vi "main 1.0.vi"() -> ()   [LabVIEW 2020]
uses:
  subvi/Newport ESP301/Newport ESP301.lvlib
  subvi/sp_manip.llb/sp_manip_lib.lvlib
  subvi/sp_manip.llb/tcp_gateway.lvlib
  subvi/PHOIBOS/DEFINITIONS/DEF_dev_type.ctl
  subvi/PHOIBOS/DEFINITIONS/DEF_dev_state.ctl
  <vilib>/Utility/file.llb/Write Delimited Spreadsheet (DBL).vi
  <vilib>/Analysis/NI_AALBase.lvlib
  <vilib>/Analysis/1siggen.llb/Ramp Pattern by Samples.vi
  <vilib>/Analysis/NI_AALPro.lvlib
  <vilib>/Analysis/_algsub.llb/Real Vector Norm.vi
  subvi/ZaberTSeries/ZaberTSeries.lvlib
  <vilib>/DAQmx/create/channels.llb/DAQmx Create Channel (DI-Digital Input).vi
  <vilib>/Utility/file.llb/Read Delimited Spreadsheet (string).vi
  <vilib>/Utility/file.llb/Write Delimited Spreadsheet (string).vi
panel:
  out "Pics L":i32=100
  out "Waveform Chart":dbl(graph)
  out "G2 X":cluster{dbl[], "Ramp Pattern":dbl[]}(graph)
  in  "reset every n pics":bool
  in  "pics2avg":i32=50
  in  "abort acq.":bool
  out "G2 Y":cluster{dbl[], "Ramp Pattern":dbl[]}(graph)={[0.0, 0.0, 0.0, 0.0, 0.0, 0.0, 0.0, 0.0, 0.0, 0.0, 0.0, 0.0, 0.0, 0.0, 0.0, 0.0, 0.0, 0.0, 0.0, 0.0, 0.0, 0.0, 0.0, 0.0, 0.0, 0.0, 0.0, 0.0, 0.0, 0.0, 0.0, 0.0, 0.0, 0.0, 0.0, 0.0, 0.0, 0.0, 0.0, 0.0, 0.0, 0.0, 0.0, 0.0, 0.0, 0.0, 0.0, 0.0, 0.0, 0.0, 0.0, 0.0, 0.0, 0.0, 0.0, 0.0, 0.0, 0.0, 0.0, 0.0, 0.0, 0.0, 0.0, 0.0, 0.0, 0.0, 0.0, 0.0, 0.0, 0.0, 0.0, 0.0, 0.0, 0.0, 0.0, 0.0, 0.0, 0.0, 0.0, 0.0, 0.0, 0.0, 0.0, 0.0, 0.0, 0.0, 0.0, 0.0, 0.0, 0.0, 0.0, 0.0, 0.0, 0.0, 0.0, 0.0, 0.0, 0.0, 0.0, 0.0, 0.0, 0.0, 0.0, 0.0, 0.0, 0.0, 0.0, 0.0, 0.0, 0.0, 0.0, 0.0, 0.0, 0.0, 0.0, 0.0, 0.0, 0.0, 0.0, 0.0, 0.0, 0.0, 0.0, 0.0, 0.0, 0.0, 0.0, 0.0, 0.0, 0.0, 0.0, 0.0, 0.0, 0.0, 0.0, 0.0, 0.0, 0.0, 0.0, 0.0, 0.0, 0.0, 0.0, 0.0, 0.0, 0.0, 0.0, 0.0, 0.0, 0.0, 0.0, 0.0, 0.0, 0.0, 0.0, 0.0, 0.0, 0.0, 0.0, 0.0, 0.0, 0.0, 0.0, 0.0, 0.0, 0.0, 0.0, 0.0, 0.0, 0.0, 0.0, 0.0, 0.0, 0.0, 0.0, 0.0, 0.0, 0.0, 0.0, 0.0, 0.0, 0.0, 0.0, 0.0, 0.0, 0.0, 0.0, 0.0, 0.0, 0.0, 0.0, 0.0, 0.0, 0.0, 0.0, 0.0, 0.0, 0.0, 0.0, 0.0, 0.0, 0.0, 0.0, 0.0, 0.0, 0.0, 0.0, 0.0, 0.0, 0.0, 0.0, 0.0, 0.0, 0.0, 0.0, 0.0, 0.0, 0.0, 0.0, 0.0, 0.0, 0.0, 0.0, 0.0, 0.0, 0.0, 0.0, 0.0, 0.0, 0.0, 0.0, 0.0, 0.0, 0.0, 0.0, 0.0, 0.0, 0.0, 0.0, 0.0, 0.0, 0.0, 0.0, 0.0, 0.0, 0.0, 0.0, 0.0, 0.0, 0.0, 0.0, 0.0, 0.0, 0.0, 0.0, 0.0], "Ramp Pattern"=[0.0, 1.003921568627451, 2.007843137254902, 3.011764705882353, 4.015686274509804, 5.019607843137255, 6.023529411764706, 7.027450980392157, 8.031372549019608, 9.035294117647059, 10.03921568627451, 11.04313725490196, 12.047058823529412, 13.050980392156863, 14.054901960784314, 15.058823529411764, 16.062745098039215, 17.066666666666666, 18.070588235294117, 19.07450980392157, 20.07843137254902, 21.08235294117647, 22.08627450980392, 23.090196078431372, 24.094117647058823, 25.098039215686274, 26.101960784313725, 27.105882352941176, 28.109803921568627, 29.113725490196078, 30.11764705882353, 31.12156862745098, 32.12549019607843, 33.129411764705885, 34.13333333333333, 35.13725490196079, 36.141176470588235, 37.14509803921569, 38.14901960784314, 39.15294117647059, 40.15686274509804, 41.16078431372549, 42.16470588235294, 43.168627450980395, 44.17254901960784, 45.1764705882353, 46.180392156862744, 47.1843137254902, 48.188235294117646, 49.1921568627451, 50.19607843137255, 51.2, 52.20392156862745, 53.207843137254905, 54.21176470588235, 55.21568627450981, 56.219607843137254, 57.22352941176471, 58.227450980392156, 59.23137254901961, 60.23529411764706, 61.23921568627451, 62.24313725490196, 63.247058823529414, 64.25098039215686, 65.25490196078431, 66.25882352941177, 67.26274509803922, 68.26666666666667, 69.27058823529411, 70.27450980392157, 71.27843137254902, 72.28235294117647, 73.28627450980392, 74.29019607843138, 75.29411764705883, 76.29803921568627, 77.30196078431372, 78.30588235294118, 79.30980392156863, 80.31372549019608, 81.31764705882352, 82.32156862745099, 83.32549019607843, 84.32941176470588, 85.33333333333333, 86.33725490196079, 87.34117647058824, 88.34509803921569, 89.34901960784313, 90.3529411764706, 91.35686274509804, 92.36078431372549, 93.36470588235294, 94.3686274509804, 95.37254901960785, 96.37647058823529, 97.38039215686274, 98.3843137254902, 99.38823529411765, 100.3921568627451, 101.39607843137254, 102.4, 103.40392156862745, 104.4078431372549, 105.41176470588235, 106.41568627450981, 107.41960784313726, 108.4235294117647, 109.42745098039215, 110.43137254901961, 111.43529411764706, 112.43921568627451, 113.44313725490196, 114.44705882352942, 115.45098039215686, 116.45490196078431, 117.45882352941176, 118.46274509803922, 119.46666666666667, 120.47058823529412, 121.47450980392156, 122.47843137254903, 123.48235294117647, 124.48627450980392, 125.49019607843137, 126.49411764705883, 127.49803921568628, 128.50196078431372, 129.50588235294117, 130.50980392156862, 131.51372549019607, 132.51764705882354, 133.521568627451, 134.52549019607844, 135.52941176470588, 136.53333333333333, 137.53725490196078, 138.54117647058823, 139.54509803921567, 140.54901960784315, 141.5529411764706, 142.55686274509804, 143.5607843137255, 144.56470588235294, 145.5686274509804, 146.57254901960783, 147.57647058823528, 148.58039215686276, 149.5843137254902, 150.58823529411765, 151.5921568627451, 152.59607843137255, 153.6, 154.60392156862744, 155.6078431372549, 156.61176470588236, 157.6156862745098, 158.61960784313726, 159.6235294117647, 160.62745098039215, 161.6313725490196, 162.63529411764705, 163.6392156862745, 164.64313725490197, 165.64705882352942, 166.65098039215687, 167.65490196078431, 168.65882352941176, 169.6627450980392, 170.66666666666666, 171.6705882352941, 172.67450980392158, 173.67843137254903, 174.68235294117648, 175.68627450980392, 176.69019607843137, 177.69411764705882, 178.69803921568626, 179.7019607843137, 180.7058823529412, 181.70980392156864, 182.71372549019608, 183.71764705882353, 184.72156862745098, 185.72549019607843, 186.72941176470587, 187.73333333333332, 188.7372549019608, 189.74117647058824, 190.7450980392157, 191.74901960784314, 192.75294117647059, 193.75686274509803, 194.76078431372548, 195.76470588235293, 196.7686274509804, 197.77254901960785, 198.7764705882353, 199.78039215686275, 200.7843137254902, 201.78823529411764, 202.7921568627451, 203.79607843137254, 204.8, 205.80392156862746, 206.8078431372549, 207.81176470588235, 208.8156862745098, 209.81960784313725, 210.8235294117647, 211.82745098039214, 212.83137254901962, 213.83529411764707, 214.8392156862745, 215.84313725490196, 216.8470588235294, 217.85098039215686, 218.8549019607843, 219.85882352941175, 220.86274509803923, 221.86666666666667, 222.87058823529412, 223.87450980392157, 224.87843137254902, 225.88235294117646, 226.8862745098039, 227.89019607843136, 228.89411764705883, 229.89803921568628, 230.90196078431373, 231.90588235294118, 232.90980392156862, 233.91372549019607, 234.91764705882352, 235.92156862745097, 236.92549019607844, 237.9294117647059, 238.93333333333334, 239.93725490196078, 240.94117647058823, 241.94509803921568, 242.94901960784313, 243.95294117647057, 244.95686274509805, 245.9607843137255, 246.96470588235294, 247.9686274509804, 248.97254901960784, 249.9764705882353, 250.98039215686273, 251.98431372549018, 252.98823529411766, 253.9921568627451, 254.99607843137255, 256.0]}
  out "ETA":timestamp=timestamp(3548856288.832348 s since 1904-01-01) format="%<%H:%M:%S>T"
  out "acq. imgs":i32=100
  out "snap_prog":dbl(slide)=1.0 scale=0.0..1.0
  in  "BasePath":path=path "Z:/PESdata"
  in  "cam_liveavg":bool caption="live average"
  out "cam_fps":dbl=19.997871297693028 caption="FPS" format="%.1g"
  out "sideimg":dbl[][](graph)
  out "RunNumber":u16=53
  out "sum":dbl format="%#.2g"
  out "max":dbl
  out "mainimg":dbl[][](graph)
  out "ESP_con?":bool=TRUE caption="ESP301"
  out "phoib_con?":bool caption="PHOIBOS"
  out "manip_con?":bool caption="manipulator"
  out "cam_con?":bool caption="camera"
  in  "main_close":bool=TRUE
  in  "Tab Control":enum32{"live", "1D scan", "devices"}(tab)
  in  "ESP_opent0file":bool
  in  "mirr_rel":i32=100 caption="relative [steps]"
  in  "mirr_Y-":bool
  in  "mirr_Y+":bool
  in  "mirr_X+":bool
  in  "mirr_X-":bool
  in  "manip_deltas":dbl[](array[numeric])=[0.0, 0.0, 0.0, 0.0, 10.0, 0.0] caption="delta" format="%#.5g"
  in  "aq.mode":enum32{"Radio Selection 1", "Radio Selection 2"}(radio)=enum."Radio Selection 2"
  in  "dark avg":i32=100
  in  "cam_avgs":i32=100 caption="N"
  in  "ESP_delta":dbl caption="relative [mm]"
  in  "ESP_-":bool
  in  "ESP_+":bool
  in  "ESP_go":bool
  in  "ESP_dest_t":dbl=-29399.00509438431 caption="[fs]"
  in  "ESP_dest":dbl=26.8972 caption="[mm]"
  in  "ESP_set_t0":bool
  in  "phoib_I_6s":dbl=3200.0
  in  "phoib_I_5s":dbl=1650.0
  in  "phoib_I_4s":dbl=4.558
  in  "phoib_I_3s":dbl=-7.0
  in  "phoib_I_2s":dbl=20.0
  in  "phoib_I_1s":dbl=22.3
  in  "phoib_standby":bool
  in  "phoib_set":bool
  out "phoib_I_6":dbl caption="Screen Voltage"
  out "phoib_I_5":dbl caption="Detctor Voltage"
  out "phoib_I_4":dbl caption="Work Function"
  out "phoib_I_3":dbl caption="Coil Current"
  out "phoib_I_2":dbl caption="Pass Energy"
  out "phoib_I_1":dbl caption="Kinetic Energy"
  out "Saved Positions":string[][](table)=[["ertwertwert", "-2.299945", "-2.030214", "38.900024", "50.000762", "0.000887", "-97.998082"], ["uztgugt", "-14.999451", "-13.638894", "442.380066", "13.998380", "-1.893758", "-76.305838"], ["asdf", "-14.999451", "-13.638894", "442.380066", "13.998380", "-1.893758", "-76.305838"], ["test3", "-14.999451", "-13.638894", "441.380066", "13.998380", "-1.893758", "-76.305838"]]
  in  "Save Pos":bool
  in  "Load":bool
  in  "Delete":bool
  in  "ManipRel +":bool
  in  "ManipRel -":bool
  in  "Move Abs":bool
  in  "stop manip":bool
  in  "dest":dbl[](array[numeric])=[-2.6172862113166087, -0.009888298846365134, 68.5008544921875, -46.36280498847848, 1.1073518432055398, -218.56360350415366] caption="destination" format="%#.5g"
  out "axis":string[](array[string])=["x", "y", "z", "polar", "tilt", "azimut"]
  out "pos":dbl[](array[numeric])=[-2.6172862113166087, -0.009888298846365134, 68.5008544921875, -46.363686276590336, 11.108982061941884, -218.56360350415366] caption="position" format="%.5f"
  in  "ana_mode":T1(ring)=enum."WideAngleMode"
  in  "ana_voltrange":enum16{"3.5kV", "1.5kV", "400V", "100V", "10V"}(ring)=enum."400V"
  out "ESP_pos":dbl caption="Position"
  out "ESP_delay":dbl=-179438.80362727473 caption="Delay"
  out "ESP_t0":dbl=26.8972 caption="Time Zero @"
  out "phoib_I_7":dbl caption="Conversion Voltage"
  in  "phoib_I_7s":dbl=-16.0
  in  "phoib_I_8s":dbl=0.0039
  in  "phoib_I_9s":dbl=0.0039
  out "phoib_I_8":dbl caption="FD1"
  out "phoib_I_9":dbl caption="FD2"
  in  "gain":bool
  in  "cam_exp":u32=50 caption="exposure [ms]"
  in  "binning":u16(ring)=2 items=["X 1", "X 2", "X 4", "X 8"]
  in  "cam_dark?":bool=TRUE caption="subtract dark?"
  in  "cam_dark":bool
  in  "cam_saveimg":bool
  in  "e-size":u8
  in  "lower threshold":i32=50
  in  "count?":bool
  in  "ROI Left":i32=1
  in  "ROI Right":i32=43
  in  "ROI Top":i32=1
  in  "ROI Bottom":i32=33
  out "moving?":bool[](array[boolean])
  out "mirr_posX":i32=-64 caption="X"
  out "mirr_posY":i32=-2601 caption="Y"
  out "anglegraph":dbl[][](graph)
  out "energygraph":dbl[][](graph)
  out "intensitygraph":cluster{"Array":dbl[], "Intensity Chart":dbl[]}(graph)={"Array"=[-150.0, -100.0, -50.0, -35.0, -20.0, -5.0, 10.0, 25.0, 40.0, 55.0, 70.0, 85.0, 100.0, 115.0, 130.0, 145.0, 160.0, 175.0, 190.0, 205.0, 220.0, 235.0, 250.0, 265.0, 280.0, 295.0, 310.0, 325.0, 340.0, 355.0, 370.0, 385.0, 400.0, 415.0, 430.0, 445.0, 460.0, 475.0, 490.0, 500.0], "Intensity Chart"=[132631.53314285746, 170205.20628571414, 433170.403142859, 542203.6841176483, 639885.119117649, 741255.8358823535, 780214.1202941145, 723815.9523529416, 738264.4005882328, 646980.995000003, 619153.8497058817, 580506.1526470593, 562378.3302941191, 555223.7020588254, 508731.1714705883, 492875.9105882345, 439033.47882352717, 441388.6888235267, 404170.4791176476, 373711.9720588232, 381822.3105882356, 359925.29558823496, 351860.5002941196, 337771.13382353063, 318137.1158823533, 311051.49176470697, 306919.1505882367, 294871.7938235281, 279774.3152941182, 259292.23117647012, 259622.08852941066, 250686.10264705878, 265393.0864705881, 240220.9167647057, 248753.78529411796, 229977.45470588165, 224752.04058823473, 222836.25676470587, 224622.8149999999, 221137.03852941145]}
  in  "scan_selector":enum32{"delay", "manip", "mirror", "volt"}(tab)
  in  "scan_manip_setstart":bool
  in  "scan_manip_start":dbl[](array[numeric])=[-2.6172862113166087, -0.009888298846365134, 68.5008544921875, -46.363686276590336, 11.108982061941884, -218.56360350415366] caption="start position" format="%#.5g"
  in  "scan_manip_deltas":dbl[](array[numeric])=[0.0, 0.0, 0.0, 0.0, 10.0, 0.0] caption="direction vector\n(gets normed)" format="%#.5g"
  in  "scan_mirr_start":i32[](array[numeric])=[-64, -2601]
  in  "scan_mirr_deltas":i32[](array[numeric])=[0, 0, 0, 0, 10, 0] caption="direction vector\n(gets normed)"
  in  "scan_mirr_setstart":bool
  in  "scan_volt_parameter":string(combo)="Kinetic Energy"
  in  "meas_iter":i32=60 caption="Iterations"
  out "duration [HH:MM:SS]":dbl=55.62603882380894 format="%<%H:%M:%S>t"
  out "disk [MB]":dbl=1327.2
  out "RAM [MB]":dbl=22.12
  out "total steps":i32=2400
  out "measpoints":i32=40
  in  "load delay table":bool
  in  "scan_go":bool
  in  "waypoints":string[][](table)=[["-150", "50"], ["-50", "15"], ["500", ""]]
  out "ETA":timestamp=timestamp(3548967985.4284124 s since 1904-01-01) format="%<%H:%M:%S>T"
  in  "stop":bool
  out "scan":dbl(slide)=0.125 scale=0.0..1.0
  out "iteration":dbl(slide)=0.5833333333333334 scale=0.0..1.0
  out "current scan":i32=5
  out "current iteration":i32=35
  in  "mirr_init":bool
  in  "mirr_release":bool
  in  "mirr_Y#":u8=2
  in  "manip_init":bool
  in  "manip_release":bool
  in  "phoib_init":bool
  in  "phoib_release":bool
  in  "ESP_init":bool
  in  "ESP_release":bool
  in  "ESP301 VISA":refnum<visa-resource-name>="COM8"
  in  "board number":i32
  in  "cam_init":bool
  in  "cam_release":bool
  out "cam_error":errorcluster
  out "phoib_error":errorcluster
  out "state":T2 items=["Off"=-1, "Standby"=0, "On"=1]
  in  "ESP Axis":i32=1 min=1 max=3
  out "error out":errorcluster={"status"=TRUE, "code"=-1073807339, "source"="VISA Read in Newport ESP301.lvlib:Write Command and Read.vi->Newport ESP301.lvlib:Read Actual Position.vi->main 1.0 alpha.vi"}
  out "error out 2":errorcluster={"status"=TRUE, "code"=1, "source"="TCP Write in sp_manip_lib.lvlib:sp_manip_disconnect.vi->main 1.0 alpha.vi"}
  out "mirr_Error":errorcluster={"status"=FALSE, "code"=1073676418, "source"="VISA Close in ZaberTSeries.lvlib:Close.vi->main 1.0 alpha.vi"}
  in  "mirr_VISA":refnum<visa-resource-name>="COM7"
  in  "mirr_X#":u8=1
  in  "Operating mode\nHP & QE / HS & DiCam Pro":u32=1
  in  "Frame trigger \n(High Performance and QE only)":u16
  # "camera"
  # "analyzer"
  # "manipulator"
  # "aquisition"
  # "delay stage"
  # "mirror"
  # "Position"
  # "Destination"
  # "- no settings -"
  # "waypoints are absolute values"
  # "X\nY\nZ\npolar\ntilt\nazimut"
  # "waypoint \"0\" is start position"
  # "X\nY"
  # "waypoint \"0\" is start position"
  # "waypoints are absolute values"
  # "camera"
  # "phoibos"
  # "ESP301"
  # "manipulator"
  # "mirror"
  # "0 = sequential\n1 = simultaneous"
  # "0 = internal\n1 = external rising\n2 = external falling"
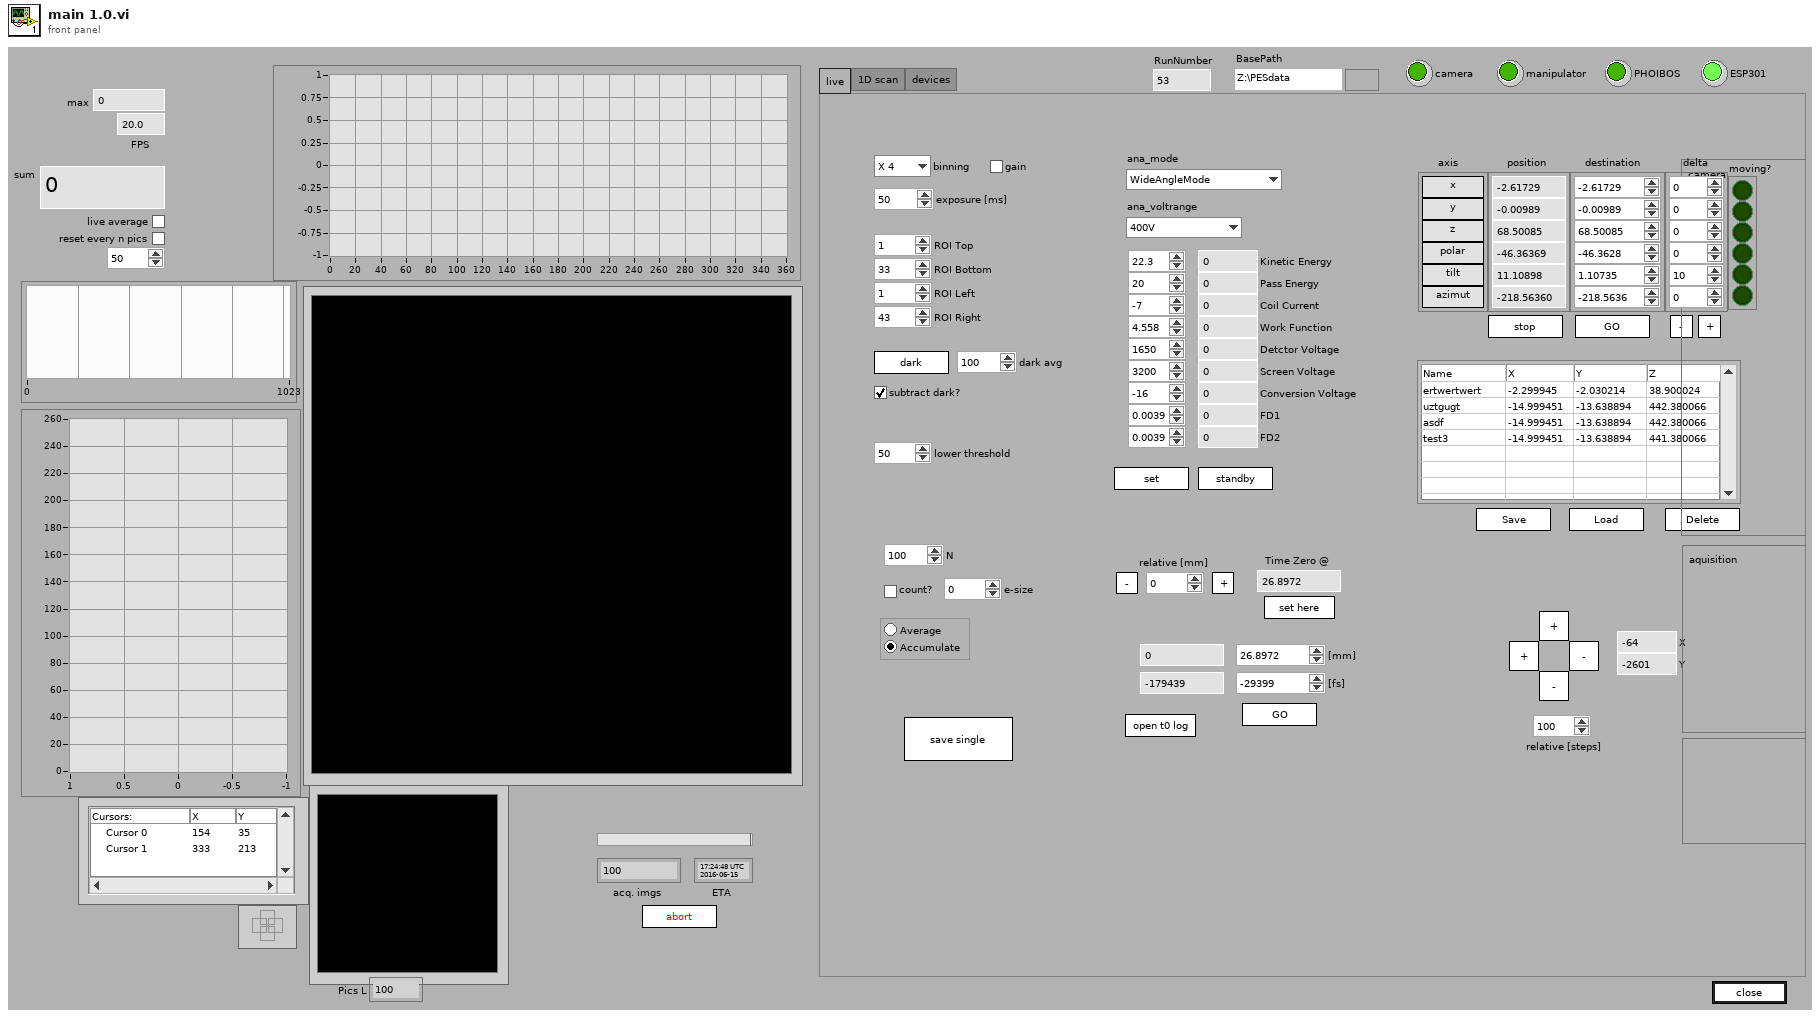
[diagram p1: front panel]
types:
  T1 = enum16{"HighMagnification", "MediumMagnification", "LowMagnification", "HighAngularDispersion", "MediumAngularDispersion", "LowAngularDispersion", "WideAngleMode", "LargeArea", "MediumArea", "SmallArea", "HighMagnification2", "SmallArea2", "ImagingMode"}
  T2 = typedef "DEF_dev_state.ctl" = i32
  T3 = cluster{"queue out":refnum<queue>, "queue out":refnum<queue>, "queue out":refnum<queue>, "queue out":refnum<queue>, "queue out":refnum<queue>}
  T4 = typedef "LVCursorListTypeDef.ctl" = cluster{"Name":string, "Color":u32, "Style":u8, "Point Style":u8, "Name Visible":bool, "Allow Drag":bool, "Cursor Mode":u32, "Plot":i32, "Index":i32, "Position":cluster{"X":dbl, "Y":dbl}, "X Scale":u32, "Y Scale":u32, "Watch Plots":i32[], "Watch All Plots":bool, "Plot Area":i32, "Label Offset":cluster{"X":dbl, "Y":dbl}}[]
  T5 = cluster{"Camera type":u32, "Operating mode\nHP & QE / HS & DiCam Pro ":u32, "Frame trigger \n(High Performance and QE only)":u16, "Sequence trigger":u16, "Low Light\n(QE only)":bool, "Gain":bool, "Horzontal\nbinning":u16, "Vertical\nbinning ":u16, "ROI Left":i32, "ROI Right":i32, "ROI Top":i32, "ROI Bottom":i32}
  T6 = cluster{"Name":string, "Color":u32, "Style":u8, "Point Style":u8, "Name Visible":bool, "Allow Drag":bool, "Cursor Mode":u32, "Plot":i32, "Index":i32, "Position":cluster{"X":dbl, "Y":dbl}, "X Scale":u32, "Y Scale":u32, "Watch Plots":i32[], "Watch All Plots":bool, "Plot Area":i32, "Label Offset":cluster{"X":dbl, "Y":dbl}}
  T7 = cluster{"mirr_X#":u8, "Command":u8, dbl, "Response Count":i32}
  T8 = cluster{"mirr_Y#":u8, "Command":u8, dbl, "Response Count":i32}
  T9 = cluster{i32, "Command":u8, i32, "Response Count":i32}
  T10 = cluster{"Axis_Name":string, "Axis_Type":string, "Axis_Position":dbl, "continous":bool, "moving":bool}[]
  T11 = typedef "DEF_dev_type.ctl" = enum32{"devA (analyzer)", "devD (detector)"}
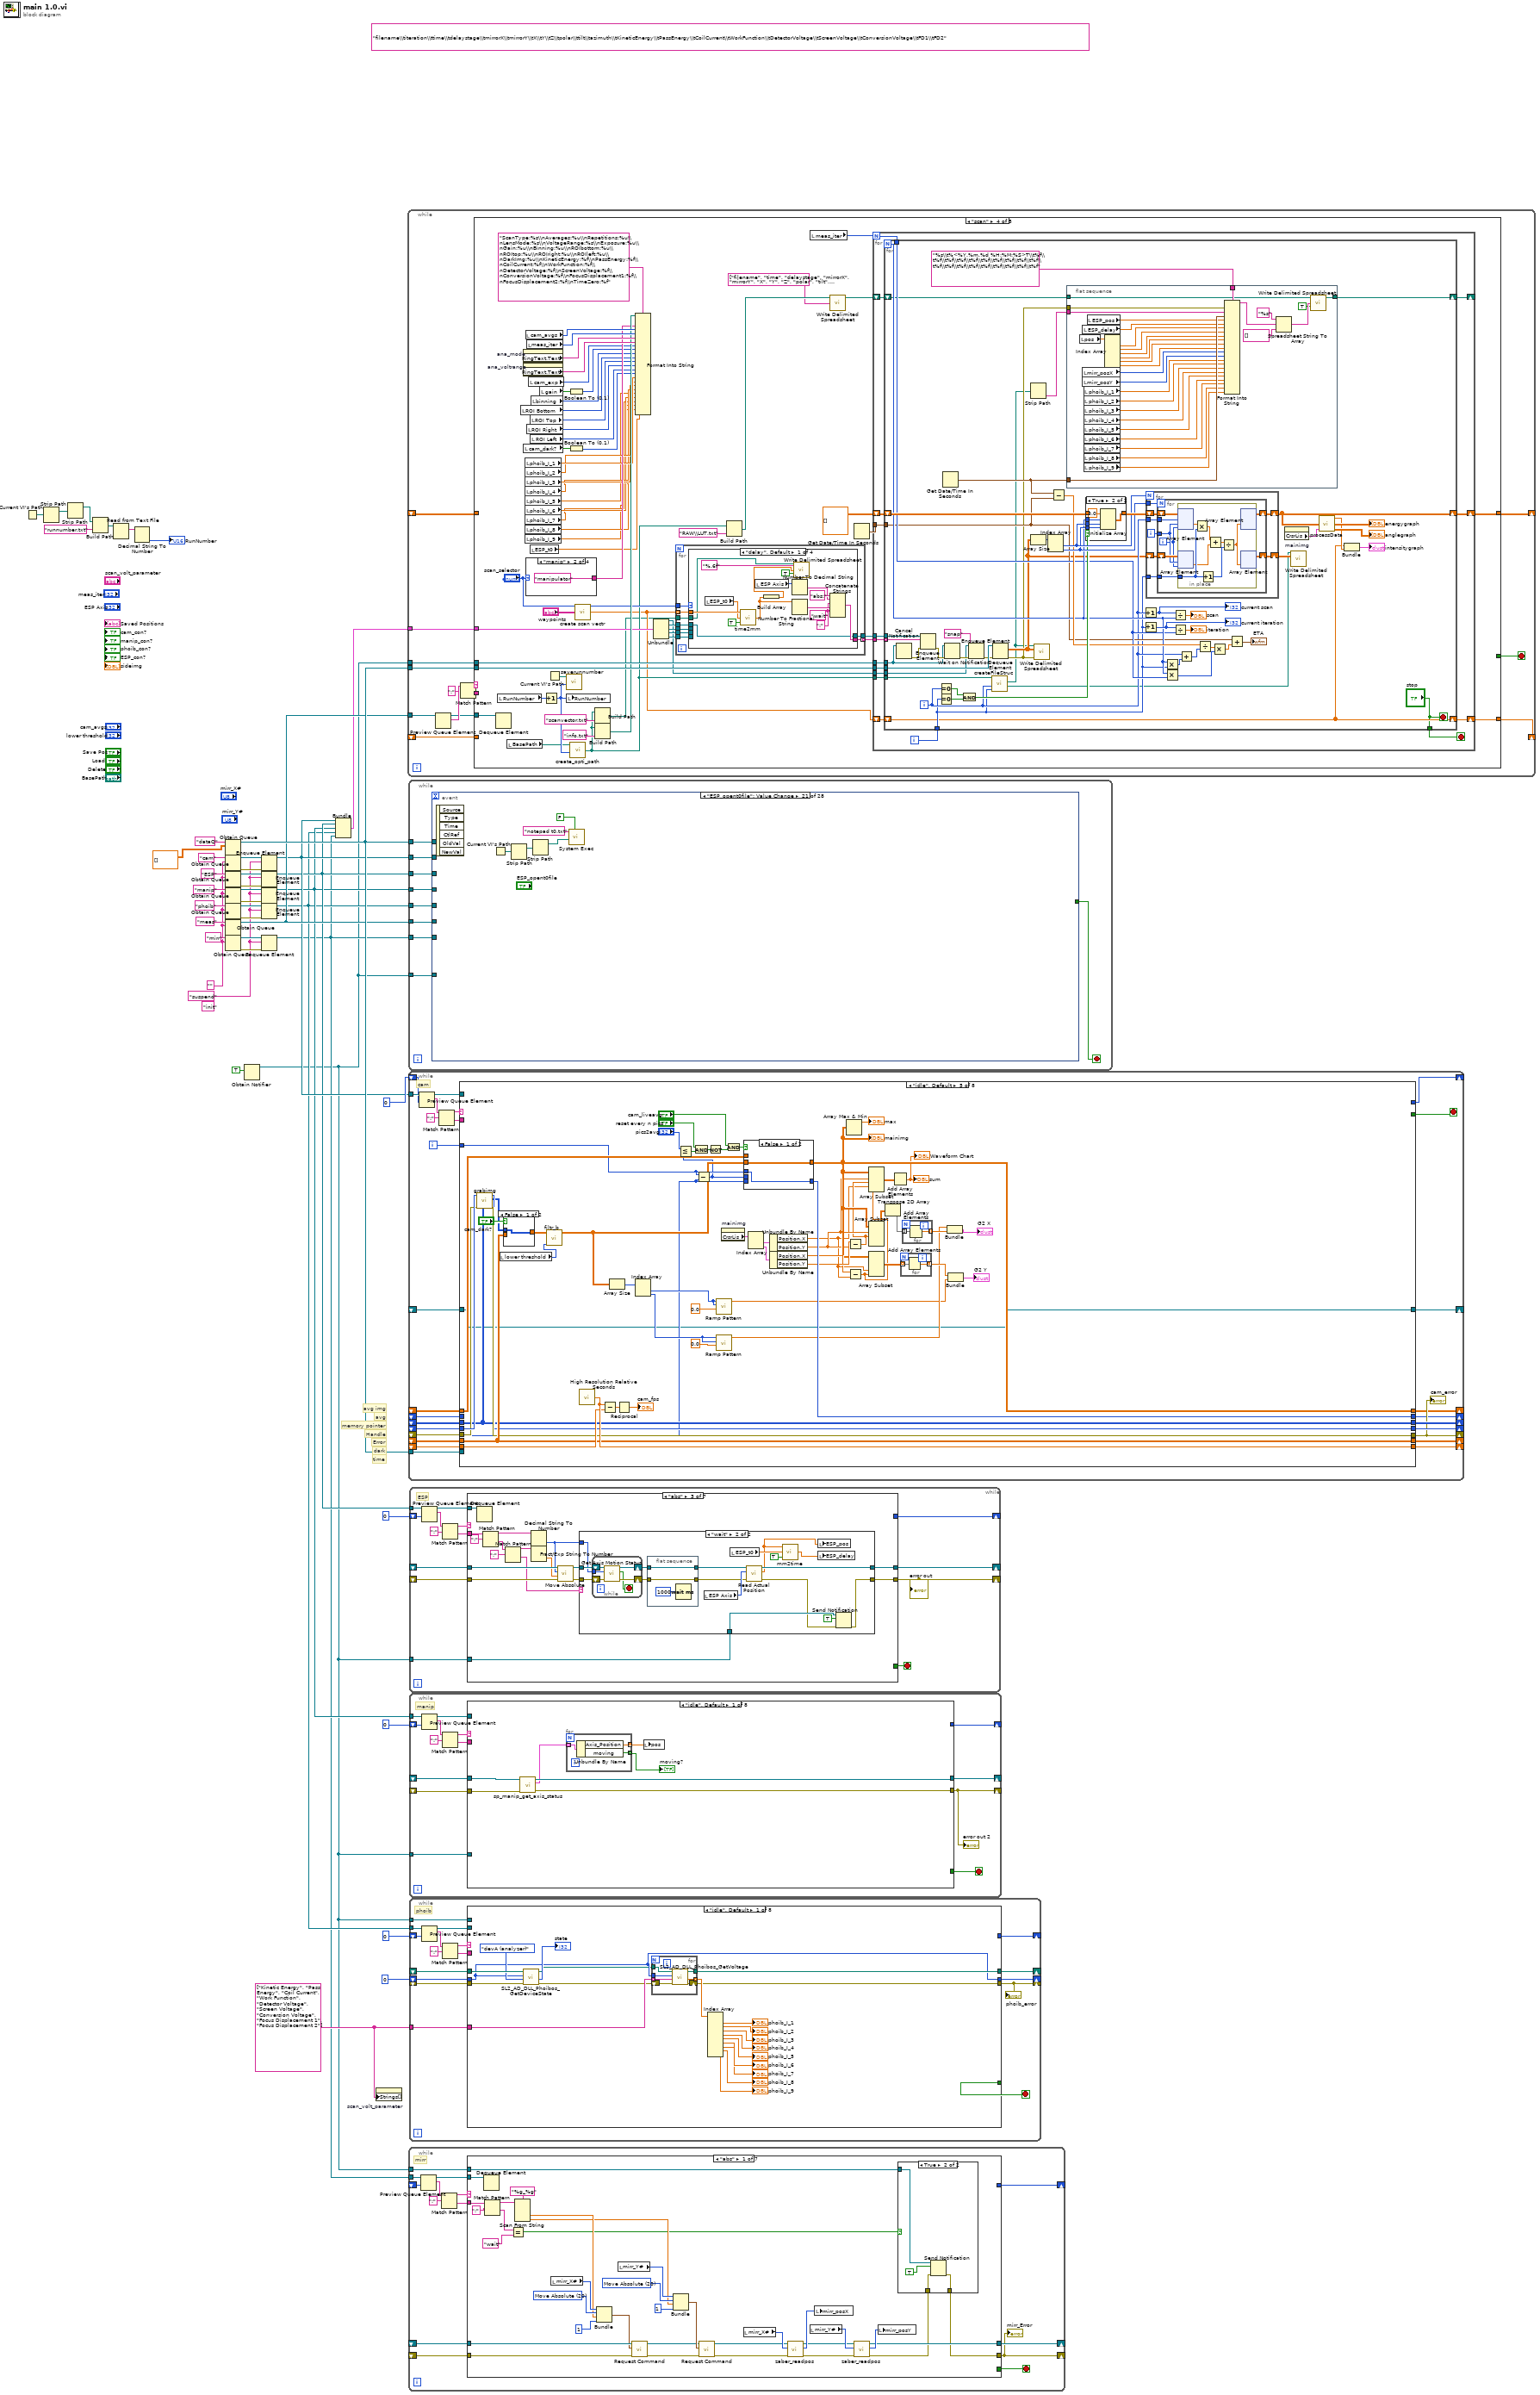
[diagram p0: block diagram]
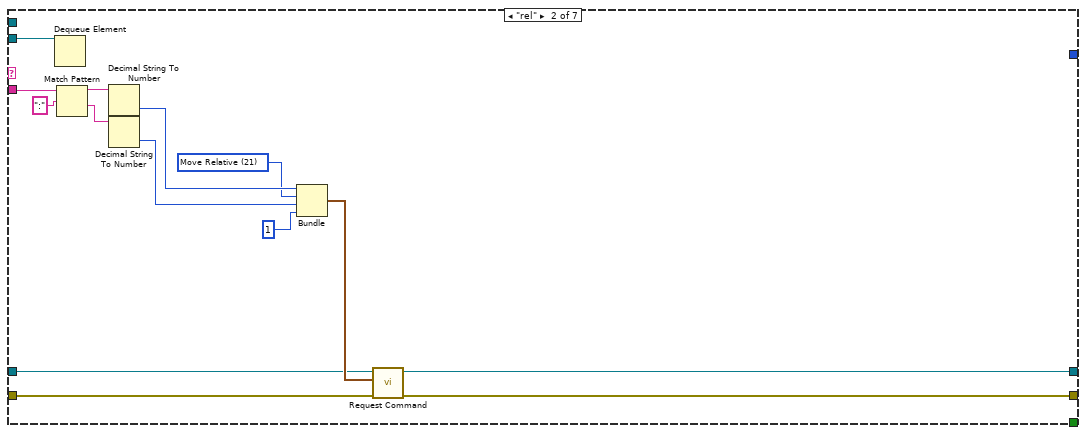
[diagram p3: hidden frame]
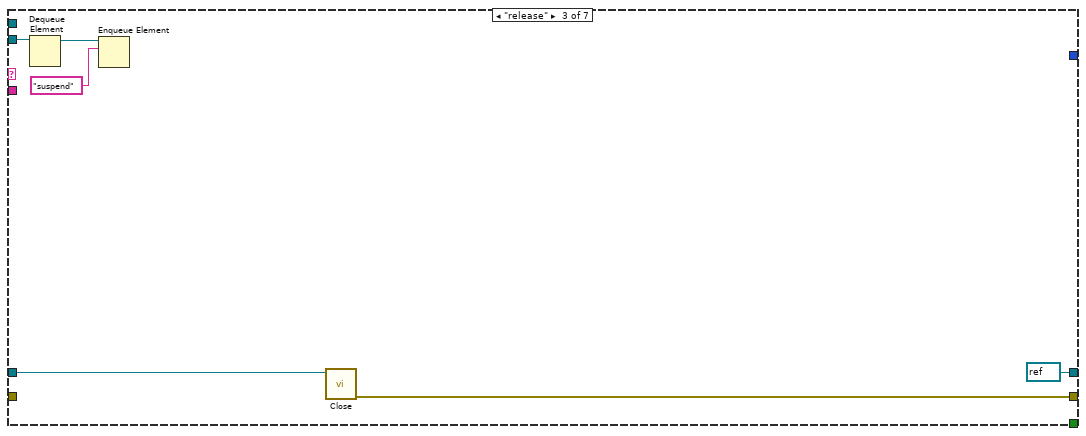
[diagram p4: hidden frame]
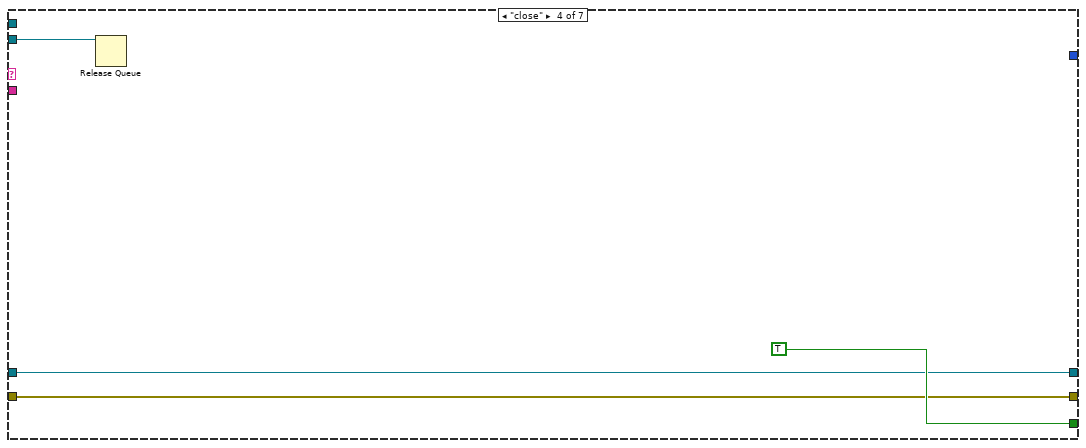
[diagram p5: hidden frame]
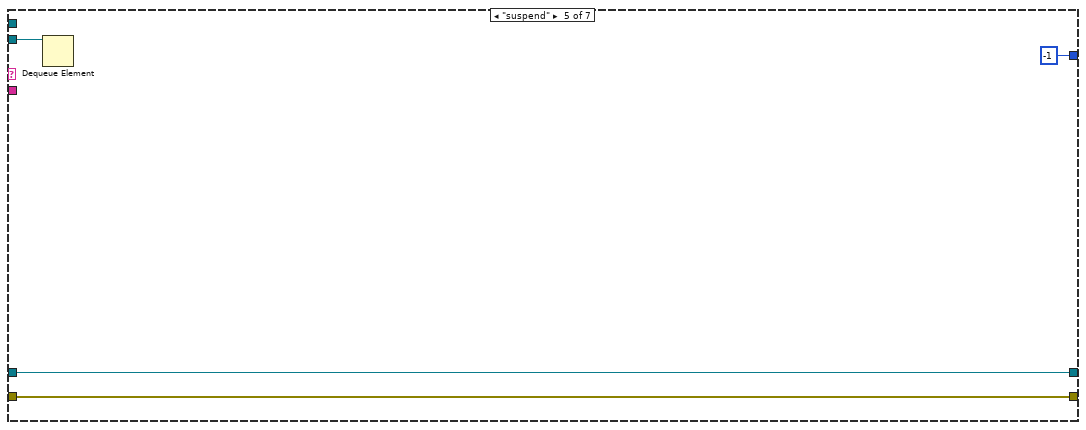
[diagram p6: hidden frame]
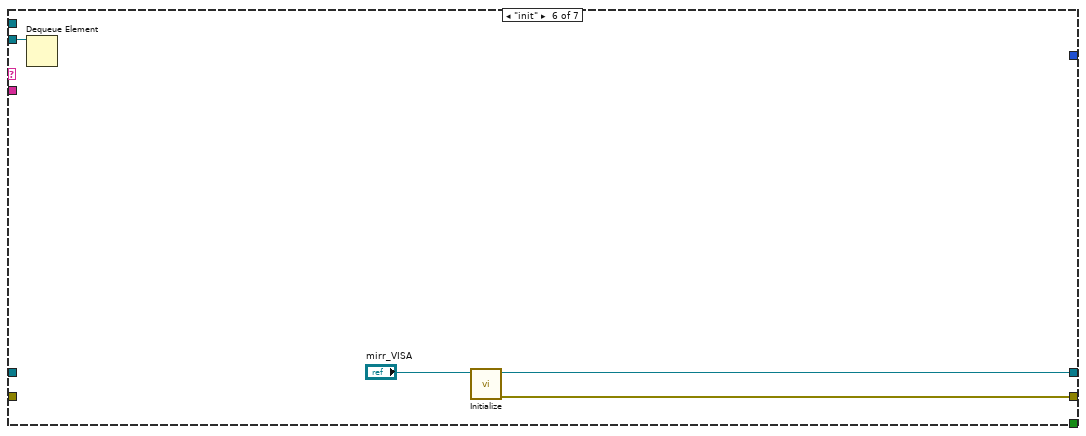
[diagram p7: hidden frame]
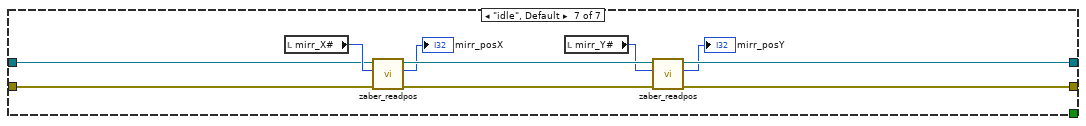
[diagram p8: hidden frame]
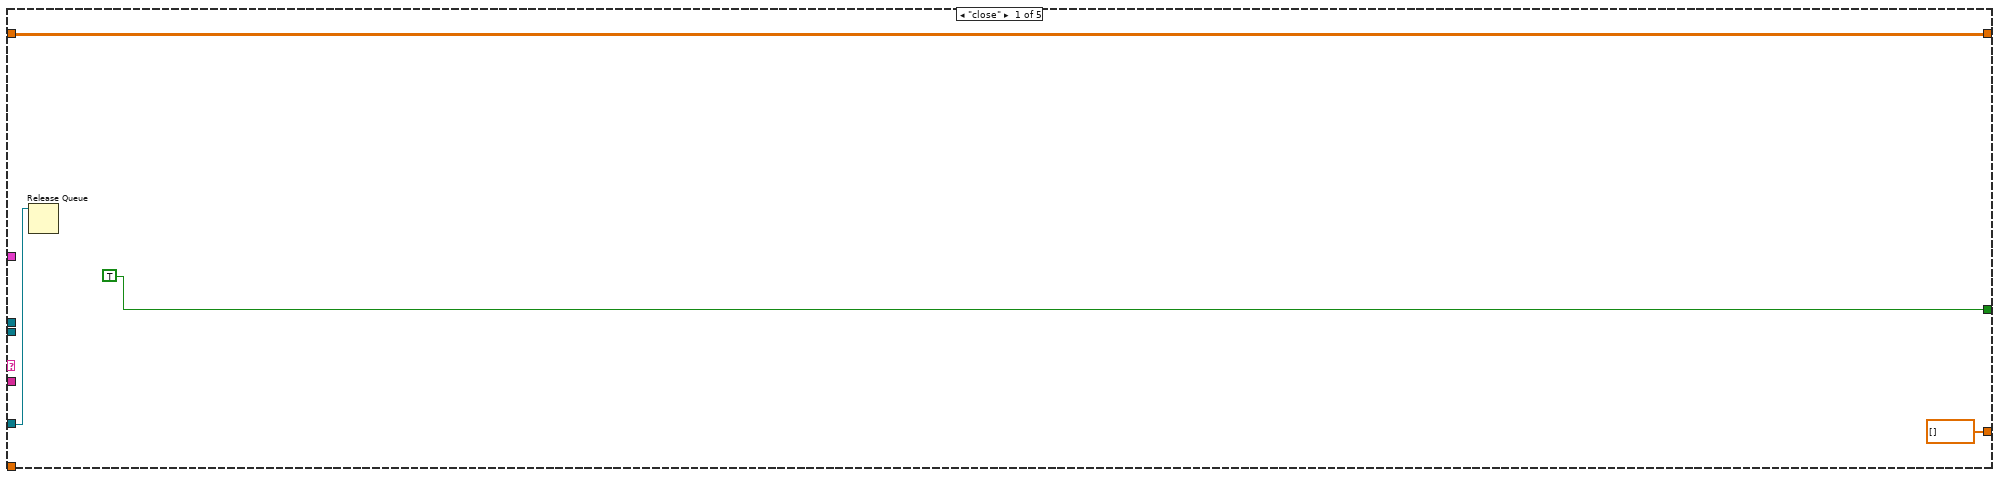
[diagram p9: hidden frame]
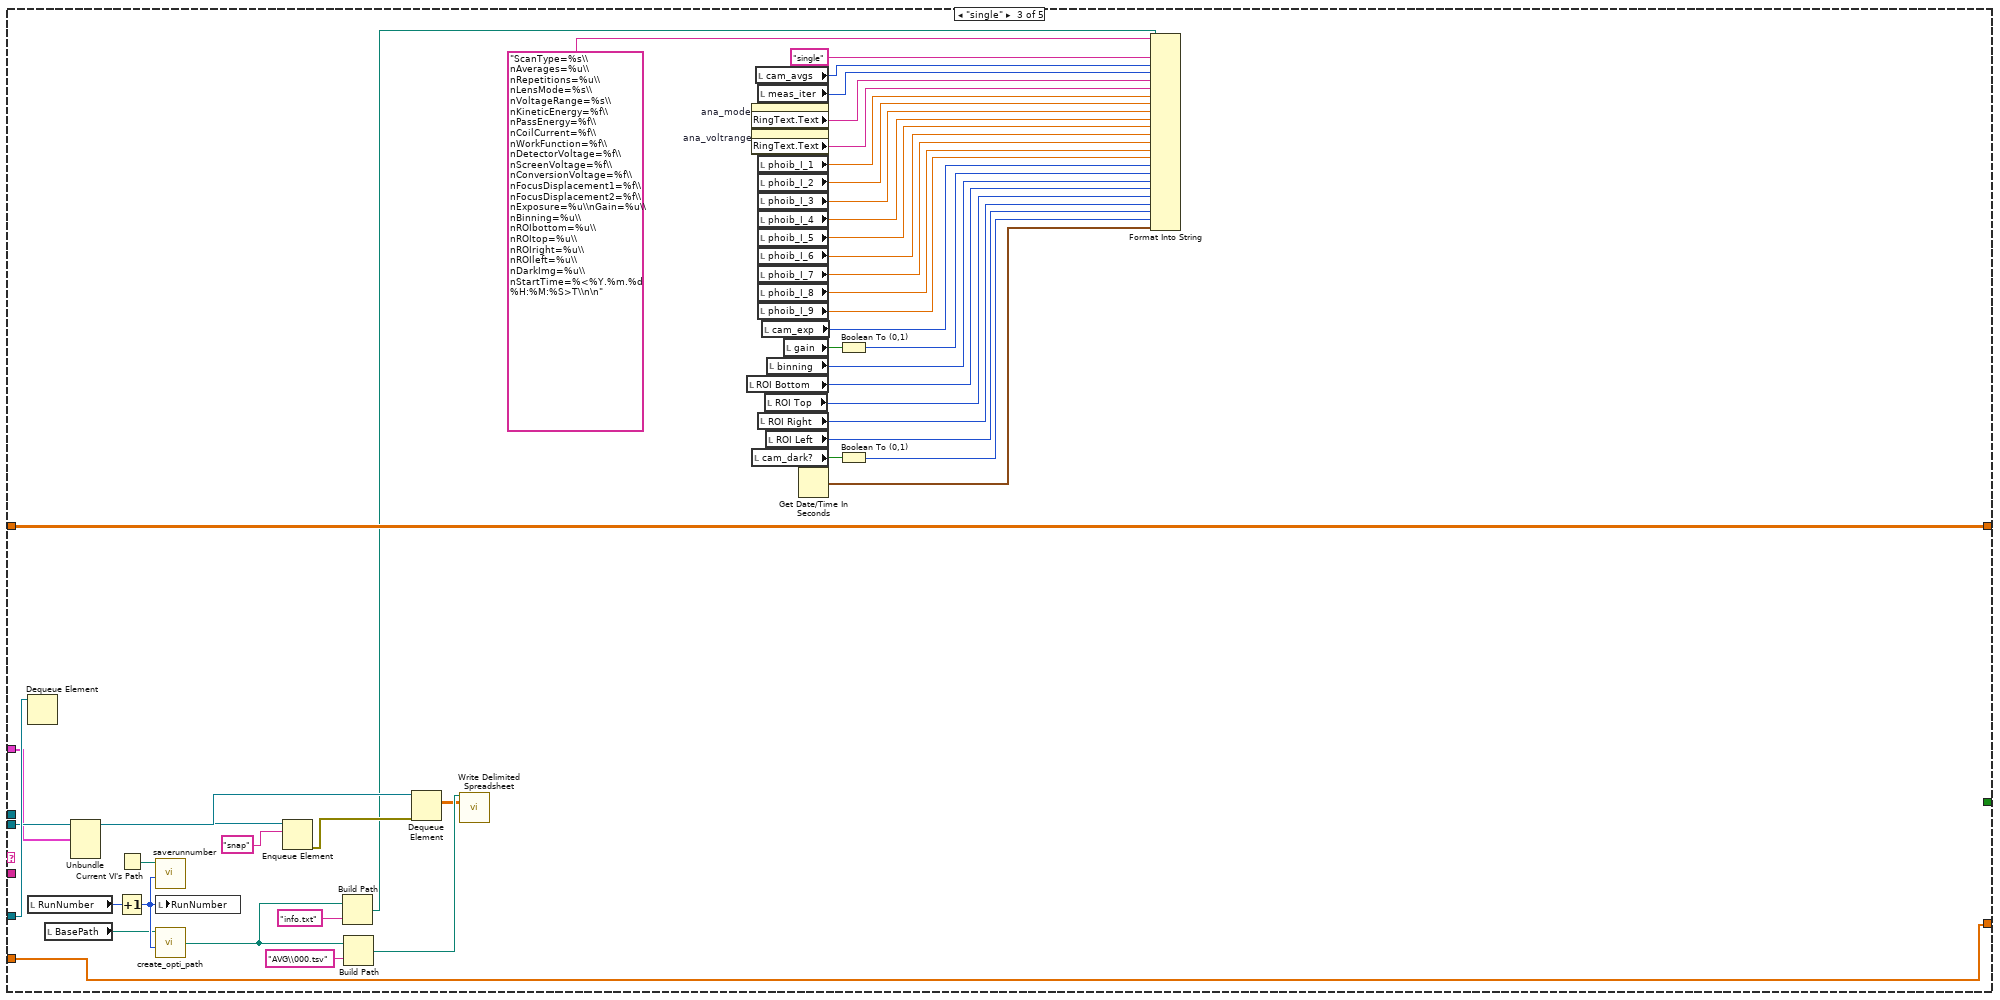
[diagram p11: hidden frame]
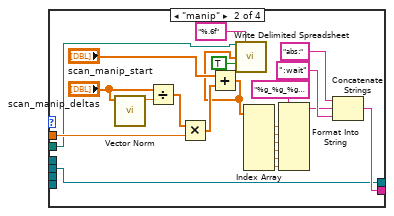
[diagram p12: hidden frame]
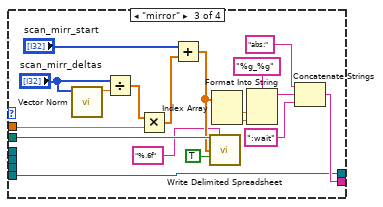
[diagram p13: hidden frame]
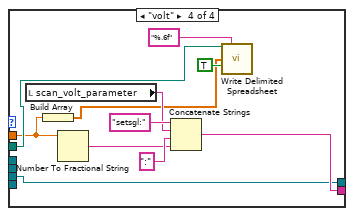
[diagram p14: hidden frame]
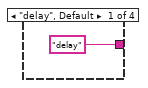
[diagram p15: hidden frame]
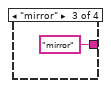
[diagram p16: hidden frame]
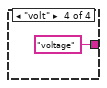
[diagram p17: hidden frame]
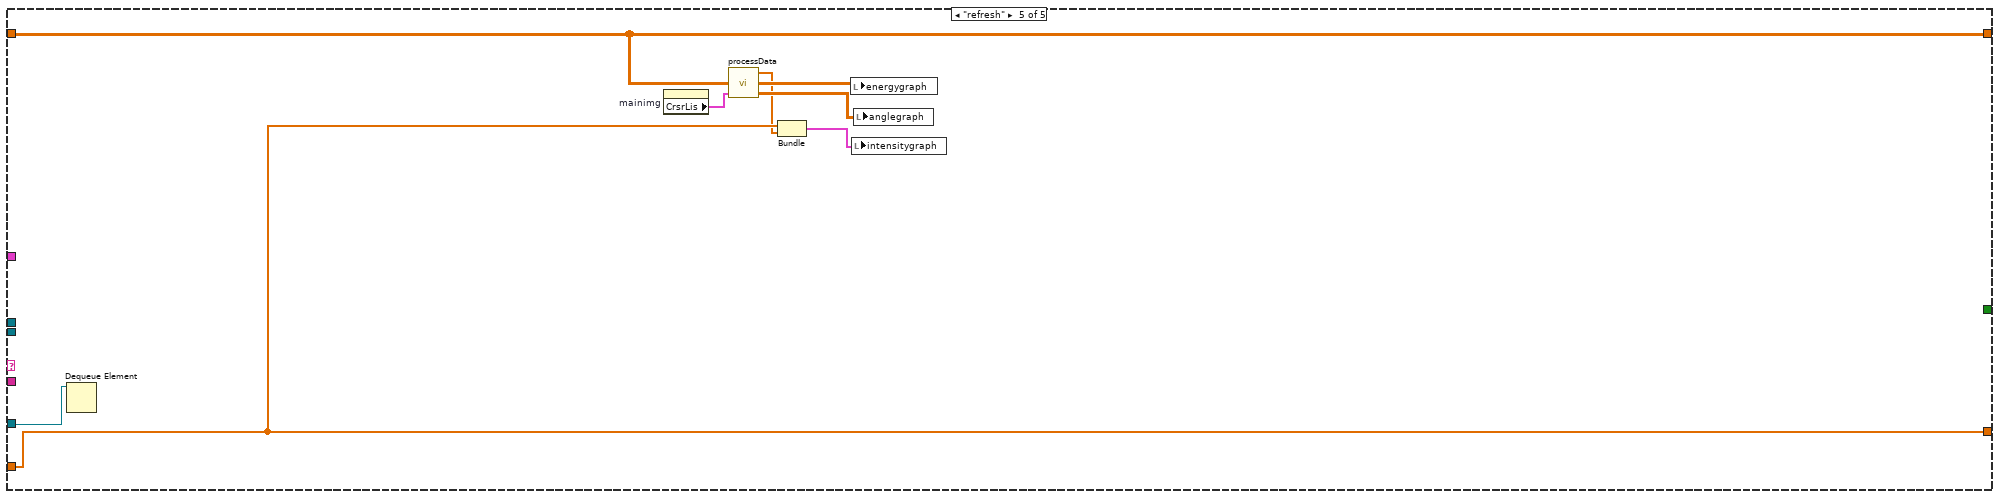
[diagram p19: hidden frame]
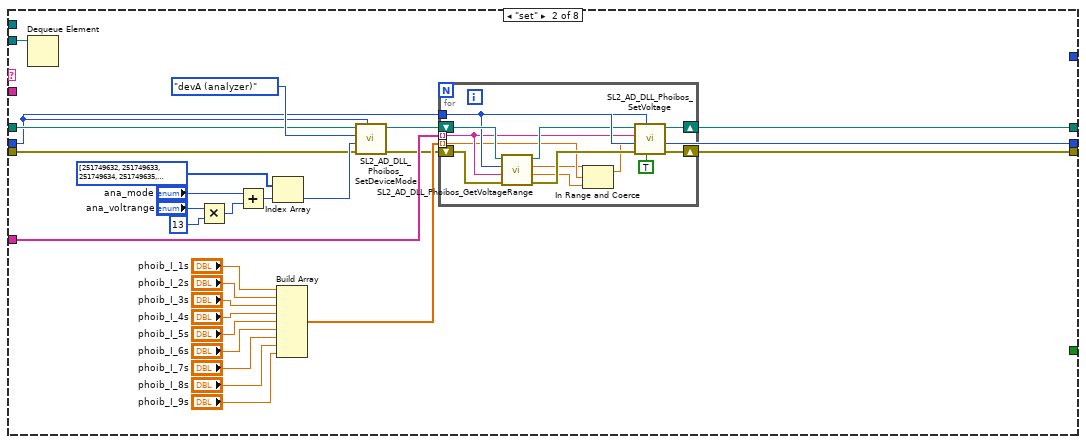
[diagram p20: hidden frame]
diagram:
  (unwired) "filename\\titeration\\ttime\\tdelaystage\\tmirrorX\\tmirrorY\\tX\\tY\\tZ\\tpolar\\ttilt\\tazimuth\\tKineticEnergy\\tPassEnergy\\tCoilCurrent\\tWorkFunction\\tDetectorVoltage\\tScreenVoltage\\tConversionVoltage\\tFD1\\tFD2"
  w9 = string[] ["Kinetic Energy", "Pass Energy", "Coil Current", "Work Function", "Detector Voltage", "Screen Voltage", "Conversion Voltage", "Focus Displacement 1", "Focus Displacement 2"]
  (unwired) "init" ("name (unnamed)")
  w1 = "suspend" ("name (unnamed)")
  w2 = "" ("name (unnamed)")
  # "avg img"
  # "avg"
  # "time"
  # "dark"
  # "Error"
  # "Handle"
  # "memory pointer"
  n1 = Current VI's Path() -> (path=w17:path)
  n2 = Strip Path(path=w17) -> (stripped path=w21:path)  [unwired: 1 out]
  n3 = Strip Path(path=w21) -> (stripped path=w22:path)  [unwired: 1 out]
  n4 = Build Path(base path=w22, name or relative path="runnumber.txt") -> (appended path=w19:path)
  n5 = Read from Text File(file (use dialog)=w19) -> (text=w20:string)  [unwired: 3 in, 3 out]
  n6 = Decimal String To Number(string=w20) -> (number=→"RunNumber":i32)  [unwired: 2 in, 1 out]
  n7 = Obtain Queue(name (unnamed)="dataQ", element data type=dbl[][] []) -> (queue out=w23:refnum<queue>)  [unwired: 3 in, 2 out]
  n8 = Obtain Queue(name (unnamed)="cam", element data type=w2) -> (queue out=w42:refnum<queue>, error out=w41:errorcluster)  [unwired: 3 in, 1 out]
  n9 = Obtain Queue(name (unnamed)="ESP", element data type=w2) -> (queue out=w39:refnum<queue>, error out=w40:errorcluster)  [unwired: 3 in, 1 out]
  n10 = Obtain Queue(name (unnamed)="manip", element data type=w2) -> (queue out=w36:refnum<queue>, error out=w35:errorcluster)  [unwired: 3 in, 1 out]
  n11 = Obtain Queue(name (unnamed)="phoib", element data type=w2) -> (queue out=w33:refnum<queue>, error out=w34:errorcluster)  [unwired: 3 in, 1 out]
  n12 = Obtain Queue(name (unnamed)="meas", element data type=w2) -> (queue out=w16:refnum<queue>)  [unwired: 3 in, 2 out]
  n13 = Obtain Queue(name (unnamed)="mirr", element data type=w2) -> (queue out=w7:refnum<queue>, error out=w6:errorcluster)  [unwired: 3 in, 1 out]
  n14 = Obtain Notifier(notification data type=TRUE) -> (notifier out=w3:refnum<notifier>)  [unwired: 3 in, 2 out]
  n15 = Enqueue Element(queue=w42, element=w1, error in (no error)=w41) -> (queue out=w14:refnum<queue>)  [unwired: 1 in, 2 out]
  n16 = Enqueue Element(queue=w39, element=w1, error in (no error)=w40) -> (queue out=w13:refnum<queue>)  [unwired: 1 in, 2 out]
  n17 = Enqueue Element(queue=w36, element=w1, error in (no error)=w35) -> (queue out=w12:refnum<queue>)  [unwired: 1 in, 2 out]
  n18 = Enqueue Element(queue=w33, element=w1, error in (no error)=w34) -> (queue out=w11:refnum<queue>)  [unwired: 1 in, 2 out]
  n19 = Enqueue Element(queue=w7, element=w1, error in (no error)=w6) -> (queue out=w4:refnum<queue>)  [unwired: 1 in, 2 out]
  n20 = Bundle("queue out"=w14, "queue out"=w13, "queue out"=w12, "queue out"=w11, "queue out"=w4) -> (w15:T3)  [unwired: 1 in]
  n21 = property on="scan_volt_parameter" class="CmbBox"("Strings[]"=w9) -> ()  [unwired: 2 in, 2 out]
  n22 = while {
    tunnel: w23 -> [w57]
    tunnel: w16 -> [w54]
    tunnel: w15 -> [w50]
    shift-right: [w48] -> _
    shift-left: _ -> [w47]
    tunnel: w3 -> [w46]
    shift-right: [w45] -> _
    shift-left: _ -> [w44]
    stop <- w49 stop-if-true
    n23 = Preview Queue Element(queue=w54) -> (queue out=w51:refnum<queue>, element=w56:string)  [unwired: 2 in, 2 out]
    n24 = Match Pattern(string=w56, regular expression=":") -> (before substring=w53:string, after substring=w52:string)  [unwired: 1 in, 2 out]
    n25 = case shown="\"scan\"" w53 {
      tunnel: w57 -> [_ _ w106 w158 _]
      tunnel: w52 -> [_ _ _ _ _]
      tunnel: w51 -> [w61 _ w107 w154 w375]
      tunnel: [TRUE _ _ _ _] -> w49
      tunnel: w50 -> [_ _ w94 w134 _]
      tunnel: [w59 w63 w92 w156 w381] -> w48
      tunnel: w47 -> [w59 w63 w92 _ w381]
      tunnel: w46 -> [_ _ _ w155 _]
      tunnel: [dbl[] [] ("Array") w62 w64 w120 w377] -> w45
      tunnel: w44 -> [_ w62 w64 _ w377]
      frame "close" {
        n26 = Release Queue(queue=w61) -> ()  [unwired: 2 in, 3 out]
      }
      frame "idle", Default {
      }
      frame "single" {
        n27 = Dequeue Element(queue=w107) -> ()  [unwired: 2 in, 4 out]
        n28 = local read "RunNumber"() -> (w101:u16)
        n29 = local read "BasePath"() -> (w102:path)
        n30 = Unbundle(w94) -> ("queue out"=w93:refnum<queue>)  [unwired: 4 out]
        n31 = Increment(x=w101) -> (x+1=w103:u16)
        n32 = Current VI's Path() -> (path=w100:path)
        n33 = call "saverunnumber.vi"("RunNumber"=w103, "VI path"=w100) -> ()  [unwired: 10 in]
        n34 = local write "RunNumber"(w103) -> ()
        n35 = call "create_opti_path.vi"("RunNumber"=w103, "base path"=w102) -> ("Path"=w96:path)  [unwired: 2 in]
        n36 = Enqueue Element(queue=w93, element="snap" ("string")) -> (error out=w104:errorcluster)  [unwired: 2 in, 2 out]
        n37 = Build Path(base path=w96, name or relative path="info.txt") -> (appended path=w65:path)
        n38 = Build Path(base path=w96, name or relative path="AVG\\000.tsv") -> (appended path=w98:path)
        n39 = Dequeue Element(queue=w106, error in (no error)=w104) -> (element=w95:dbl[][])  [unwired: 1 in, 3 out]
        n40 = call-poly <vilib>:"Write Delimited Spreadsheet.vi"("file path (dialog if empty)"=w98, "2D data"=w95) -> ()  [unwired: 12 in, 2 out]
        n41 = local read "ROI Bottom"() -> (w72:i32)
        n42 = property on="ana_mode" class="Enum (strict)"() -> ("RingText.Text"=w87:string)  [unwired: 2 in, 2 out]
        n43 = property on="ana_voltrange" class="Enum (strict)"() -> ("RingText.Text"=w86:string)  [unwired: 2 in, 2 out]
        n44 = local read "cam_dark?"() -> (w68:bool)
        n45 = local read "cam_avgs"() -> (w89:i32)
        n46 = local read "meas_iter"() -> (w88:i32)
        n47 = local read "phoib_I_1"() -> (w85:dbl)
        n48 = local read "phoib_I_2"() -> (w84:dbl)
        n49 = local read "phoib_I_3"() -> (w83:dbl)
        n50 = local read "phoib_I_4"() -> (w82:dbl)
        n51 = local read "phoib_I_5"() -> (w81:dbl)
        n52 = local read "phoib_I_6"() -> (w80:dbl)
        n53 = local read "phoib_I_7"() -> (w79:dbl)
        n54 = local read "phoib_I_8"() -> (w78:dbl)
        n55 = local read "phoib_I_9"() -> (w77:dbl)
        n56 = local read "ROI Right"() -> (w70:i32)
        n57 = local read "cam_exp"() -> (w76:u32)
        n58 = local read "ROI Top"() -> (w71:i32)
        n59 = local read "ROI Left"() -> (w69:i32)
        n60 = local read "binning"() -> (w73:u16)
        n61 = local read "gain"() -> (w75:bool)
        n62 = Get Date/Time In Seconds() -> (seconds since 1Jan1904=w66:timestamp)
        n63 = Boolean To (0,1)(Boolean=w75) -> (0, 1=w74:i16)
        n64 = Boolean To (0,1)(Boolean=w68) -> (0, 1=w67:i16)
        n65 = Format Into String(format string="ScanType=%s\\nAverages=%u\\nRepetitions=%u\\nLensMode=%s\\nVoltageRange=%s\\nKineticEnergy=%f\\nPassEnergy=%f\\nCoilCurrent=%f\\nWorkFunction=%f\\nDetectorVoltage=%f\\nScreenVoltage=%f\\nConversionVoltage=%f\\nFocusDisplacement1=%f\\nFocusDisplacement2=%f\\nExposure=%u\\nGain=%u\\nBinning=%u\\nROIbottom=%u\\nROItop=%u\\nROIright=%u\\nROIleft=%u\\nDarkImg=%u\\nStartTime=%<%Y.%m.%d %H:%M:%S>T\\n\n", initial string=w65, "single" ("input 1"), w89, w88, w87, w86, w85, w84, w83, w82, w81, w80, w79, w78, w77, w76, w74, w73, w72, w71, w70, w69, w67, w66) -> ()  [unwired: 1 in, 2 out]
      }
      frame "scan" {
        n66 = Dequeue Element(queue=w154) -> ()  [unwired: 2 in, 4 out]
        n67 = local read "RunNumber"() -> (w163:u16)
        n68 = local read "BasePath"() -> (w164:path)
        n69 = local read "ROI Bottom"() -> (w140:i32)
        n70 = property on="ana_mode" class="Enum (strict)"() -> ("RingText.Text"=w149:string)  [unwired: 2 in, 2 out]
        n71 = property on="ana_voltrange" class="Enum (strict)"() -> ("RingText.Text"=w148:string)  [unwired: 2 in, 2 out]
        n72 = local read "cam_dark?"() -> (w146:bool)
        n73 = local read "phoib_I_1"() -> (w118:dbl)
        n74 = local read "phoib_I_2"() -> (w117:dbl)
        n75 = local read "phoib_I_3"() -> (w116:dbl)
        n76 = local read "phoib_I_4"() -> (w115:dbl)
        n77 = local read "phoib_I_5"() -> (w114:dbl)
        n78 = local read "phoib_I_6"() -> (w113:dbl)
        n79 = local read "phoib_I_7"() -> (w112:dbl)
        n80 = local read "phoib_I_8"() -> (w111:dbl)
        n81 = local read "phoib_I_9"() -> (w110:dbl)
        n82 = local read "cam_avgs"() -> (w151:i32)
        n83 = case shown="\"manip\"" "scan_selector" {
          tunnel: ["delay" ("input 1") "manipulator" ("input 1") "mirror" ("input 1") "voltage" ("input 1")] -> w144
          frame "delay", Default {
          }
          frame "manip" {
          }
          frame "mirror" {
          }
          frame "volt" {
          }
        }
        n84 = local read "meas_iter"() -> (w150:i32)
        n85 = local read "ROI Right"() -> (w138:i32)
        n86 = local read "cam_exp"() -> (w143:u32)
        n87 = local read "ROI Top"() -> (w139:i32)
        n88 = local read "ESP_t0"() -> (w109:dbl)
        n89 = local read "ROI Left"() -> (w137:i32)
        n90 = local read "binning"() -> (w141:u16)
        n91 = local read "gain"() -> (w147:bool)
        n92 = Increment(x=w163) -> (x+1=w165:u16)
        n93 = Current VI's Path() -> (path=w162:path)
        n94 = call "saverunnumber.vi"("RunNumber"=w165, "VI path"=w162) -> ()  [unwired: 10 in]
        n95 = local write "RunNumber"(w165) -> ()
        n96 = Boolean To (0,1)(Boolean=w147) -> (0, 1=w142:i16)
        n97 = Boolean To (0,1)(Boolean=w146) -> (0, 1=w136:i16)
        n98 = call "create_opti_path.vi"("RunNumber"=w165, "base path"=w164) -> ("Path"=w125:path)  [unwired: 2 in]
        n99 = call "create scan vectr.vi"("Table Control"="waypoints") -> ("Array"=w119:dbl[])
        n100 = Build Path(base path=w125, name or relative path="scanvector.txt") -> (appended path=w108:path)
        n101 = Build Path(base path=w125, name or relative path="info.txt") -> (appended path=w145:path)
        n102 = Format Into String(format string="ScanType:%s\\nAverages:%u\\nRepetitions:%u\\nLensMode:%s\\nVoltageRange:%s\\nExposure:%u\\nGain:%u\\nBinning:%u\\nROIbottom:%u\\nROItop:%u\\nROIright:%u\\nROIleft:%u\\nDarkImg:%u\\nKineticEnergy:%f\\nPassEnergy:%f\\nCoilCurrent:%f\\nWorkFunction:%f\\nDetectorVoltage:%f\\nScreenVoltage:%f\\nConversionVoltage:%f\\nFocusDisplacement1:%f\\nFocusDisplacement2:%f\\nTimeZero:%f", initial string=w145, w144, w151, w150, w149, w148, w143, w142, w141, w140, w139, w138, w137, w136, w118, w117, w116, w115, w114, w113, w112, w111, w110, w109) -> ()  [unwired: 1 in, 2 out]
        n103 = Unbundle(w134) -> ("queue out"=w126:refnum<queue>, "queue out"=w133:refnum<queue>, "queue out"=w132:refnum<queue>, "queue out"=w131:refnum<queue>, "queue out"=w130:refnum<queue>)
        n104 = for {
          tunnel: w119 -> [w174] mode=indexing
          tunnel: [w173] -> w127 mode=indexing
          tunnel: [w172] -> w128
          tunnel: w133 -> [w171]
          tunnel: w132 -> [w170]
          tunnel: w131 -> [w169]
          tunnel: w130 -> [w168]
          tunnel: "scan_selector" -> [w167]
          tunnel: w108 -> [w166]
          n105 = case shown="\"delay\", Default" w167 {
            tunnel: w174 -> [w182 w209 w222 w232]
            tunnel: [w180 w197 w219 w236] -> w172
            tunnel: [w186 w198 w220 w237] -> w173
            tunnel: w171 -> [w180 _ _ _]
            tunnel: w170 -> [_ w197 _ _]
            tunnel: w169 -> [_ _ _ w236]
            tunnel: w168 -> [_ _ w219 _]
            tunnel: w166 -> [w175 w192 w216 w233]
            frame "delay", Default {
              w188 = ":" ("string")
              n106 = local read "ESP_t0"() -> (w181:dbl)
              n107 = call "time2mm.vi"("fs[1]/ps[0]"=TRUE, "Offset (mm)"=w181, "time"=w182) -> ("position (mm)"=w177:dbl)
              n108 = local read "ESP Axis"() -> (w185:i32)
              n109 = Build Array(w177) -> (w176:dbl[])
              n110 = Number To Decimal String(number=w185) -> (decimal integer string=w184:string)  [unwired: 1 in]
              n111 = Number To Fractional String(number=w177) -> (F-format string=w190:string)  [unwired: 3 in]
              n112 = call-poly <vilib>:"Write Delimited Spreadsheet.vi"("file path (dialog if empty)"=w175, "format (%.3f)"="%.6f", "1D data"=w176, "append to file? (new file:F)"=TRUE ("append to file? (F)")) -> ()  [unwired: 10 in, 2 out]
              n113 = Concatenate Strings("abs:" ("string"), w184, w188, w190, w188, "wait" ("string")) -> (w186:string)
            }
            frame "manip" {
              n114 = call-poly <vilib>:"Vector Norm.vi"("Input Vector"="scan_manip_deltas") -> ("norm"=w211:dbl)  [unwired: 9 in, 1 out]
              n115 = Divide(x="scan_manip_deltas", y=w211) -> (x/y=w210:dbl[])
              n116 = Multiply(x=w210, y=w209) -> (x*y=w195:dbl[])
              n117 = Add(x="scan_manip_start", y=w195) -> (x+y=w191:dbl[])
              n118 = call-poly <vilib>:"Write Delimited Spreadsheet.vi"("file path (dialog if empty)"=w192, "format (%.3f)"="%.6f", "1D data"=w191, "append to file? (new file:F)"=TRUE ("append to file? (F)")) -> ()  [unwired: 10 in, 2 out]
              n119 = Index Array(array=w191) -> (element #1=w200:dbl, element #2=w201:dbl, element #3=w202:dbl, element #4=w203:dbl, element #5=w204:dbl, element #6=w205:dbl)  [unwired: 6 in]
              n120 = Format Into String(format string="%g_%g_%g_%g_%g_%g", w200, w201, w202, w203, w204, w205) -> (resulting string=w207:string)  [unwired: 2 in, 1 out]
              n121 = Concatenate Strings("abs:" ("string"), w207, ":wait" ("string")) -> (w198:string)
            }
            frame "mirror" {
              n122 = call-poly <vilib>:"Vector Norm.vi"("Input Vector"="scan_mirr_deltas") -> ("norm"=w230:dbl)  [unwired: 9 in, 1 out]
              n123 = Divide(x="scan_mirr_deltas", y=w230) -> (x/y=w229:dbl[])
              n124 = Multiply(x=w229, y=w222) -> (x*y=w218:dbl[])
              n125 = Add(x="scan_mirr_start", y=w218) -> (x+y=w215:dbl[])
              n126 = call-poly <vilib>:"Write Delimited Spreadsheet.vi"("file path (dialog if empty)"=w216, "format (%.3f)"="%.6f", "1D data"=w215, "append to file? (new file:F)"=TRUE ("append to file? (F)")) -> ()  [unwired: 10 in, 2 out]
              n127 = Index Array(array=w215) -> (element #1=w225:dbl, element #2=w226:dbl)  [unwired: 2 in]
              n128 = Format Into String(format string="%g_%g", w225, w226) -> (resulting string=w228:string)  [unwired: 2 in, 1 out]
              n129 = Concatenate Strings("abs:" ("string"), w228, ":wait" ("string")) -> (w220:string)
            }
            frame "volt" {
              n130 = local read "scan_volt_parameter"() -> (w240:string)
              n131 = Build Array(w232) -> (w231:dbl[])
              n132 = Number To Fractional String(number=w232) -> (F-format string=w238:string)  [unwired: 3 in]
              n133 = Concatenate Strings("setsgl:" ("string"), w240, ":" ("string"), w238) -> (w237:string)
              n134 = call-poly <vilib>:"Write Delimited Spreadsheet.vi"("file path (dialog if empty)"=w233, "format (%.3f)"="%.6f", "1D data"=w231, "append to file? (new file:F)"=TRUE ("append to file? (F)")) -> ()  [unwired: 10 in, 2 out]
            }
          }
        }
        n135 = Build Path(base path=w125, name or relative path="RAW\\LUT.txt") -> (appended path=w123:path)
        n136 = local read "meas_iter"() -> (w159:i32)
        n137 = call-poly <vilib>:"Write Delimited Spreadsheet.vi"("file path (dialog if empty)"=w123, "1D data"=string[] ["filename", "time", "delaystage", "mirrorX", "mirrorY", "X", "Y", "Z", "polar", "tilt", "azimuth", "KineticEnergy", "PassEnergy", "CoilCurrent", "WorkFunction", "DetectorVoltage", "ScreenVoltage", "ConversionVoltage", "FD1", "FD2"]) -> ("new file path (Not A Path if cancelled)"=w122:path)  [unwired: 12 in, 1 out]
        n138 = Get Date/Time In Seconds() -> (seconds since 1Jan1904=w135:timestamp)
        n139 = for {
          N: w159 -> [w255]
          tunnel: w125 -> [w261]
          tunnel: w158 -> [w260]
          shift-right: [w258] -> w156
          shift-left: dbl[][][] [] -> [w257]
          tunnel: w155 -> [w256]
          tunnel: w135 -> [w254]
          tunnel: w128 -> [w253]
          tunnel: w127 -> [w252]
          tunnel: w126 -> [w251]
          shift-right: [w249] -> _
          shift-left: w122 -> [w250]
          shift-right: [w248] -> w120
          shift-left: w119 -> [w247]
          i -> [w259]
          stop <- w246 stop-if-true
          n140 = for {
            N -> [w286]
            tunnel: w261 -> [w280]
            tunnel: w260 -> [w310]
            tunnel: w259 -> [w278]
            shift-right: [w299] -> w258
            shift-left: w257 -> [w306]
            tunnel: w256 -> [w301]
            tunnel: w255 -> [w285]
            tunnel: w254 -> [w283]
            tunnel: w253 -> [w274]
            tunnel: w252 -> [w273] mode=indexing
            tunnel: w251 -> [w272]
            shift-right: [w268] -> w249
            shift-left: w250 -> [w269]
            shift-right: [w264] -> w248
            shift-left: w247 -> [w264]
            tunnel: ["stop"] -> w246
            i -> [w279]
            stop <- "stop" stop-if-true
            n141 = Cancel Notification(0:w301) -> (11:w302:errorcluster)  [unwired: 1 in, 2 out]
            n142 = Enqueue Element(queue=w274, element=w273, error in (no error)=w302) -> (error out=w305:errorcluster)  [unwired: 1 in, 2 out]
            n143 = Equal To 0?(x=w279) -> (x = 0?=w309:bool)
            n144 = Equal To 0?(x=w278) -> (x = 0?=w308:bool)
            n145 = Get Date/Time In Seconds() -> (seconds since 1Jan1904=w270:timestamp)
            n146 = Wait on Notification(notifier=w301, error in (no error)=w305) -> (error out=w304:errorcluster)  [unwired: 2 in, 3 out]
            n147 = And(x=w309, y=w308) -> (x .and. y?=w307:bool)
            n148 = Enqueue Element(queue=w272, element="snap", error in (no error)=w304) -> (error out=w303:errorcluster)  [unwired: 1 in, 2 out]
            n149 = call "createFileStruc.vi"("i_iter"=w278, "i_delay"=w279, "meas_path"=w280) -> ("AVG file"=w275:path, "RAW file"=w266:path)  [unwired: 7 in]
            n150 = Dequeue Element(queue=w310, error in (no error)=w303) -> (element=w277:dbl[][], error out=w267:errorcluster)  [unwired: 1 in, 2 out]
            n151 = Strip Path(path=w266) -> (name=w265:string)  [unwired: 1 out]
            n152 = Array Size(array=w277) -> (size(s)=w314:i32[])
            n153 = call-poly <vilib>:"Write Delimited Spreadsheet.vi"("file path (dialog if empty)"=w266, "2D data"=w277, "error in (no error)"=w267) -> ()  [unwired: 11 in, 2 out]
            n154 = Index Array(array=w314) -> (element #1=w312:i32, element #2=w311:i32)  [unwired: 2 in]
            n155 = Subtract(x=w270, y=w283) -> (x-y=w289:dbl)
            n156 = flat-sequence {
              tunnel: "%s\\t%<%Y.%m.%d %H:%M:%S>T\\t%f\\t%f\\t%f\\t%f\\t%f\\t%f\\t%f\\t%f\\t%f\\t%f\\t%f\\t%f\\t%f\\t%f\\t%f\\t%f\\t%f\\t%f\\t%f" -> [w344]
              tunnel: w270 -> [w343]
              tunnel: w269 -> [w320]
              tunnel: [w319] -> w268
              tunnel: w267 -> [w316]
              tunnel: w265 -> [w315]
              frame #0 {
                n157 = local read "pos"() -> (w345:dbl[])
                n158 = local read "mirr_posX"() -> (w332:i32)
                n159 = local read "mirr_posY"() -> (w333:i32)
                n160 = local read "ESP_delay"() -> (w325:dbl)
                n161 = local read "phoib_I_1"() -> (w334:dbl)
                n162 = local read "phoib_I_2"() -> (w335:dbl)
                n163 = local read "phoib_I_3"() -> (w336:dbl)
                n164 = local read "phoib_I_4"() -> (w337:dbl)
                n165 = local read "phoib_I_5"() -> (w338:dbl)
                n166 = local read "phoib_I_6"() -> (w339:dbl)
                n167 = local read "phoib_I_7"() -> (w340:dbl)
                n168 = local read "phoib_I_8"() -> (w341:dbl)
                n169 = local read "phoib_I_9"() -> (w342:dbl)
                n170 = local read "ESP_pos"() -> (w324:dbl)
                n171 = Index Array(array=w345) -> (element #1=w326:dbl, element #2=w327:dbl, element #3=w328:dbl, element #4=w329:dbl, element #5=w330:dbl, element #6=w331:dbl)  [unwired: 6 in]
                n172 = Format Into String(format string=w344, error in=w316, w315, w343, w324, w325, w326, w327, w328, w329, w330, w331, w332, w333, w334, w335, w336, w337, w338, w339, w340, w341, w342) -> (resulting string=w322:string)  [unwired: 1 in, 1 out]
                n173 = Spreadsheet String To Array(format string="%s", spreadsheet string=w322, array type (2D Dbl)=string[] []) -> (array=w318:string[])  [unwired: 1 in]
                n174 = call-poly <vilib>:"Write Delimited Spreadsheet.vi"("file path (dialog if empty)"=w320, "1D data"=w318, "append to file? (new file:F)"=TRUE ("append to file? (F)")) -> ("new file path (Not A Path if cancelled)"=w319:path)  [unwired: 11 in, 1 out]
              }
            }
            n175 = case shown="True" w307 {
              tunnel: w286 -> [_ w351]
              tunnel: [w346 w349] -> w313
              tunnel: w306 -> [w346 _]
              tunnel: w312 -> [_ w348]
              tunnel: w311 -> [_ w347]
              frame False {
              }
              frame True {
                n176 = Initialize Array(0.0 ("element"), w351, w348, w347) -> (w349:dbl[][][])
              }
            }
            n177 = Increment(x=w279) -> (x+1=w293:i32)
            "current scan" <- w293
            n178 = Increment(x=w278) -> (x+1=w292:i32)
            "current iteration" <- w292
            n179 = for {
              N: w312 -> [_]
              tunnel: w279 -> [w358]
              shift-right: [w356] -> w299
              shift-left: w313 -> [w359]
              tunnel: w278 -> [w354]
              shift-right: [w353] -> w276
              shift-left: w277 -> [w355]
              tunnel: w311 -> [w352]
              i -> [w357]
              n180 = for {
                N: w352 -> [_]
                tunnel: w358 -> [w366]
                tunnel: w357 -> [w363]
                shift-right: [w365] -> w356
                shift-left: w359 -> [w367]
                tunnel: w354 -> [w361]
                shift-right: [w360] -> w353
                shift-left: w355 -> [w364]
                i -> [w362]
                n181 = in-place {
                  in-place-border: w361 -> [w373]
                  n182 = in-place-array #1(w367, w366, w363, w362) -> (w374:dbl)
                  n183 = in-place-array #2(w364, w363, w362) -> (w371:dbl)
                  n184 = Multiply(x=w374, y=w373) -> (x*y=w372:dbl)
                  n185 = Increment(x=w373) -> (x+1=w369:i32)
                  n186 = Add(x=w372, y=w371) -> (x+y=w370:dbl)
                  n187 = Divide(x=w370, y=w369) -> (x/y=w368:dbl)
                  n188 = in-place-array #1(w368) -> (w365:dbl[][][])  [unwired: 3 out]
                  n189 = in-place-array #2(w368) -> (w360:dbl[][])  [unwired: 2 out]
                }
              }
            }
            n190 = Multiply(x=w286, y=w278) -> (x*y=w288:i32)
            n191 = Multiply(x=w286, y=w285) -> (x*y=w282:i32)
            n192 = Divide(x=w293, y=w286) -> (x/y=→"scan":dbl)
            n193 = Divide(x=w292, y=w285) -> (x/y=→"iteration":dbl)
            n194 = Add(x=w279, y=w288) -> (x+y=w287:i32)
            n195 = Divide(x=w289, y=w287) -> (x/y=w284:dbl)
            n196 = Multiply(x=w284, y=w282) -> (x*y=w281:dbl)
            n197 = Add(x=w283, y=w281) -> (x+y=→"ETA":timestamp)
            n198 = property on="mainimg" class="IntGraph (strict)"() -> ("CrsrLis"=w298:T4)  [unwired: 2 in, 2 out]
            n199 = call-poly <vilib>:"Write Delimited Spreadsheet.vi"("file path (dialog if empty)"=w275, "2D data"=w276) -> ()  [unwired: 12 in, 2 out]
            n200 = call "processData.vi"("Cursor List"=w298, "data in"=w299) -> ("Angle Chart"=→"anglegraph":dbl[][], "Energy Chart"=→"energygraph":dbl[][], "Intensity Chart"=w295:dbl[])  [unwired: 1 in]
            n201 = Bundle("Array"=w264, "Intensity Chart"=w295) -> (→"intensitygraph":cluster{"Array":dbl[], "Intensity Chart":dbl[]})  [unwired: 1 in]
          }
        }
      }
      frame "refresh" {
        n202 = Dequeue Element(queue=w375) -> ()  [unwired: 2 in, 4 out]
        n203 = property on="mainimg" class="IntGraph (strict)"() -> ("CrsrLis"=w382:T4)  [unwired: 2 in, 2 out]
        n204 = call "processData.vi"("Cursor List"=w382, "data in"=w381) -> ("Angle Chart"=w379:dbl[][], "Energy Chart"=w380:dbl[][], "Intensity Chart"=w376:dbl[])  [unwired: 1 in]
        n205 = Bundle("Array"=w377, "Intensity Chart"=w376) -> (w378:cluster{"Array":dbl[], "Intensity Chart":dbl[]})  [unwired: 1 in]
        n206 = local write "energygraph"(w380) -> ()
        n207 = local write "intensitygraph"(w378) -> ()
        n208 = local write "anglegraph"(w379) -> ()
      }
    }
  }
  n209 = while {
    tunnel: w14 -> [w390]
    tunnel: w13 -> [w389]
    tunnel: w12 -> [w388]
    tunnel: w11 -> [w387]
    tunnel: w16 -> [w385]
    tunnel: w23 -> [w386]
    tunnel: w3 -> [w384]
    tunnel: w4 -> [w383]
    stop <- w391 stop-if-true
    n210 = event shown="[20] \"ESP_opent0file\": Value Change" {
      selector: _ -> [_ _ _ _ _ _ _ _ _ _ _ _ _ _ _ _ _ _ _ _ _ _ _ _ _ _ _ _]
      dyn-events: _ -> [_ _ _ _ _ _ _ _ _ _ _ _ _ _ _ _ _ _ _ _ _ _ _ _ _ _ _ _]
      timeout: _ -> [_ _ _ _ _ _ _ _ _ _ _ _ _ _ _ _ _ _ _ _ _ _ _ _ _ _ _ _]
      tunnel: [_ TRUE _ _ _ _ _ _ _ _ _ _ _ _ _ _ _ _ _ _ _ _ _ _ _ _ _ _] -> w391
      tunnel: w390 -> [_ w403 w416 _ _ _ _ _ w442 w444 _ _ _ _ _ _ _ _ _ _ _ _ _ _ _ _ _ _]
      tunnel: w389 -> [_ w402 _ w420 _ _ _ _ _ _ _ _ _ _ _ _ _ _ w499 _ _ w521 _ _ _ _ _ _]
      tunnel: w388 -> [_ w401 _ _ w426 _ _ _ _ _ _ _ _ _ _ w474 w489 w491 _ _ _ _ _ _ _ _ _ _]
      tunnel: w387 -> [_ w400 _ _ _ w432 w438 w439 _ _ _ _ _ _ _ _ _ _ _ _ _ _ _ _ _ _ _ _]
      tunnel: w386 -> [_ w409 _ _ _ _ _ _ _ _ _ _ _ _ _ _ _ _ _ _ _ _ _ _ _ _ _ _]
      tunnel: w385 -> [_ w399 _ _ _ _ _ _ _ _ w446 w448 _ _ _ _ _ _ _ _ _ _ _ _ _ w540 _ _]
      tunnel: w384 -> [_ w408 _ _ _ _ _ _ _ _ _ _ _ _ _ _ _ _ _ _ _ _ _ _ _ _ _ _]
      tunnel: w383 -> [_ w398 _ _ _ _ _ _ _ _ _ _ _ _ _ _ _ _ _ _ _ _ _ _ _ _ w542 w563]
      event Timeout {
        n211 = event-data() -> ()  [unwired: 1 in, 1 out]
      }
      event "main_close": Value Change {
        w404 = "close" ("element")
        w405 = "release" ("element")
        n212 = event-data() -> ()  [unwired: 1 in, 1 out]
        n213 = Flush Queue(queue=w403) -> (queue out=w397:refnum<queue>)  [unwired: 1 in, 2 out]
        n214 = Flush Queue(queue=w402) -> (queue out=w396:refnum<queue>)  [unwired: 1 in, 2 out]
        n215 = Flush Queue(queue=w401) -> (queue out=w395:refnum<queue>)  [unwired: 1 in, 2 out]
        n216 = Flush Queue(queue=w400) -> (queue out=w394:refnum<queue>)  [unwired: 1 in, 2 out]
        n217 = Flush Queue(queue=w399) -> (queue out=w393:refnum<queue>)  [unwired: 1 in, 2 out]
        n218 = Flush Queue(queue=w398) -> (queue out=w392:refnum<queue>)  [unwired: 1 in, 2 out]
        n219 = Release Notifier(notifier=w408) -> ()  [unwired: 2 in, 3 out]
        n220 = Release Queue(queue=w409) -> ()  [unwired: 2 in, 3 out]
        n221 = Enqueue Element(queue=w397, element=w405) -> (queue out=w413:refnum<queue>)  [unwired: 2 in, 2 out]
        n222 = Enqueue Element(queue=w396, element=w405) -> (queue out=w412:refnum<queue>)  [unwired: 2 in, 2 out]
        n223 = Enqueue Element(queue=w395, element=w405) -> (queue out=w411:refnum<queue>)  [unwired: 2 in, 2 out]
        n224 = Enqueue Element(queue=w394, element=w405) -> (queue out=w410:refnum<queue>)  [unwired: 2 in, 2 out]
        n225 = Enqueue Element(queue=w392, element=w405) -> (queue out=w407:refnum<queue>, error out=w406:errorcluster)  [unwired: 2 in, 1 out]
        n226 = Enqueue Element(queue=w413, element=w404) -> ()  [unwired: 2 in, 3 out]
        n227 = Enqueue Element(queue=w412, element=w404) -> ()  [unwired: 2 in, 3 out]
        n228 = Enqueue Element(queue=w411, element=w404) -> ()  [unwired: 2 in, 3 out]
        n229 = Enqueue Element(queue=w410, element=w404) -> ()  [unwired: 2 in, 3 out]
        n230 = Enqueue Element(queue=w393, element=w404) -> ()  [unwired: 2 in, 3 out]
        n231 = Enqueue Element(queue=w407, element=w404, error in (no error)=w406) -> ()  [unwired: 1 in, 3 out]
      }
      event "cam_release", "cam_init": Value Change {
        n232 = event-data() -> ()  [unwired: 1 in, 2 out]
        n233 = Select(t="init" ("name (unnamed)"), s="cam_init", f="release" ("name (unnamed)")) -> (s? t:f=w415:string)
        n234 = Enqueue Element(queue=w416, element=w415) -> ()  [unwired: 2 in, 3 out]
      }
      event "ESP_release", "ESP_init": Value Change {
        n235 = event-data() -> ()  [unwired: 1 in, 2 out]
        n236 = Select(t="init" ("name (unnamed)"), s="ESP_init", f="release" ("name (unnamed)")) -> (s? t:f=w424:string)
        n237 = Enqueue Element(queue=w420, element=w424) -> ()  [unwired: 2 in, 3 out]
      }
      event "manip_init", "manip_release": Value Change {
        n238 = event-data() -> ()  [unwired: 1 in, 2 out]
        n239 = Flush Queue(queue=w426) -> (queue out=w425:refnum<queue>)  [unwired: 1 in, 2 out]
        n240 = Select(t="init" ("name (unnamed)"), s="manip_init", f="release" ("name (unnamed)")) -> (s? t:f=w428:string)
        n241 = Enqueue Element(queue=w425, element=w428) -> ()  [unwired: 2 in, 3 out]
      }
      event "phoib_release", "phoib_init": Value Change {
        n242 = event-data() -> ()  [unwired: 1 in, 2 out]
        n243 = Flush Queue(queue=w432) -> (queue out=w431:refnum<queue>)  [unwired: 1 in, 2 out]
        n244 = Select(t="init" ("name (unnamed)"), s="phoib_init", f="release" ("name (unnamed)")) -> (s? t:f=w434:string)
        n245 = Enqueue Element(queue=w431, element=w434) -> ()  [unwired: 2 in, 3 out]
      }
      event "phoib_standby": Value Change {
        n246 = event-data() -> ()  [unwired: 1 in, 2 out]
        n247 = Enqueue Element(queue=w438, element="standby") -> ()  [unwired: 2 in, 3 out]
      }
      event "phoib_set": Value Change {
        n248 = event-data() -> ()  [unwired: 1 in, 2 out]
        n249 = Enqueue Element(queue=w439, element="set") -> ()  [unwired: 2 in, 3 out]
      }
      event "cam_dark": Value Change {
        n250 = event-data() -> ()  [unwired: 1 in, 2 out]
        n251 = Enqueue Element(queue=w442, element="dark") -> ()  [unwired: 2 in, 3 out]
      }
      event "ROI Left", "ROI Right", "ROI Top", "ROI Bottom", "cam_exp", "binning", "gain": Value Change {
        n252 = event-data() -> ()  [unwired: 1 in, 1 out]
        n253 = Enqueue Element(queue=w444, element="set") -> ()  [unwired: 2 in, 3 out]
      }
      event "cam_saveimg": Value Change {
        n254 = event-data() -> ()  [unwired: 1 in, 1 out]
        n255 = Enqueue Element(queue=w446, element="single") -> ()  [unwired: 2 in, 3 out]
      }
      event "scan_go": Value Change {
        n256 = event-data() -> ()  [unwired: 1 in, 1 out]
        n257 = Enqueue Element(queue=w448, element="scan") -> ()  [unwired: 2 in, 3 out]
      }
      event "meas_iter", "waypoints": Value Change {
        n258 = event-data() -> ()  [unwired: 1 in, 6 out]
        n259 = local read "waypoints"() -> (w458:string[][])
        n260 = local read "meas_iter"() -> (w452:i32)
        n261 = local read "binning"() -> (w455:u16)
        n262 = call "create scan vectr.vi"("Table Control"=w458) -> ("Array"=w457:dbl[])
        n263 = Index Array(array=dbl[] [8.79, 2.2, 0.553, 0.138], index=w455) -> (element=w451:dbl)
        n264 = Array Size(array=w457) -> (size(s)=w454:i32)
        "measpoints" <- w454
        n265 = Multiply(x=w454, y=w452) -> (x*y=w449:i32)
        "total steps" <- w449
        n266 = Multiply(x=w454, y=w451) -> (x*y=→"RAM [MB]":dbl)
        n267 = Multiply(x=w449, y=w451) -> (x*y=→"disk [MB]":dbl)
      }
      event "scan_manip_setstart": Value Change {
        n268 = event-data() -> ()  [unwired: 1 in, 1 out]
        n269 = local read "pos"() -> (w459:dbl[])
        n270 = local write "scan_manip_start"(w459) -> ()
      }
      event "scan_mirr_setstart": Value Change {
        n271 = event-data() -> ()  [unwired: 1 in, 1 out]
        n272 = local read "mirr_posX"() -> (w462:i32)
        n273 = local read "mirr_posY"() -> (w461:i32)
        n274 = Build Array(w462, w461) -> (w460:i32[])
        n275 = local write "scan_mirr_start"(w460) -> ()
      }
      event "Move Abs": Value Change {
        n276 = event-data() -> ()  [unwired: 1 in, 1 out]
        n277 = Index Array(array="dest") -> (element #1=w472:dbl, element #2=w471:dbl, element #3=w470:dbl, element #4=w469:dbl, element #5=w468:dbl, element #6=w467:dbl)  [unwired: 6 in]
        n278 = Format Into String(format string="%g_%g_%g_%g_%g_%g", w472, w471, w470, w469, w468, w467) -> (resulting string=w465:string)  [unwired: 2 in, 1 out]
        n279 = Concatenate Strings("abs:" ("string"), w465) -> (w464:string)
        n280 = Enqueue Element(queue=w474, element=w464) -> ()  [unwired: 2 in, 3 out]
      }
      event "ManipRel +", "ManipRel -": Value Change {
        n281 = event-data() -> ()  [unwired: 1 in, 2 out]
        n282 = Negate(x="manip_deltas") -> (-x=w477:dbl[])
        n283 = Select(t="manip_deltas", s="ManipRel +", f=w477) -> (s? t:f=w475:dbl[])
        n284 = Index Array(array=w475) -> (element #1=w481:dbl, element #2=w482:dbl, element #3=w483:dbl, element #4=w484:dbl, element #5=w485:dbl, element #6=w486:dbl)  [unwired: 6 in]
        n285 = Format Into String(format string="%g_%g_%g_%g_%g_%g", w481, w482, w483, w484, w485, w486) -> (resulting string=w488:string)  [unwired: 2 in, 1 out]
        n286 = Concatenate Strings("rel:" ("string"), w488) -> (w479:string)
        n287 = Enqueue Element(queue=w489, element=w479) -> ()  [unwired: 2 in, 3 out]
      }
      event "stop manip": Value Change {
        n288 = event-data() -> ()  [unwired: 1 in, 1 out]
        n289 = Enqueue Element(queue=w491, element="stop") -> ()  [unwired: 2 in, 3 out]
      }
      event "ESP_go": Value Change {
        w493 = ":" ("string")
        n290 = event-data() -> ()  [unwired: 1 in, 1 out]
        n291 = local read "ESP Axis"() -> (w492:i32)
        n292 = Number To Decimal String(number=w492) -> (decimal integer string=w495:string)  [unwired: 1 in]
        n293 = Number To Fractional String(number="ESP_dest") -> (F-format string=w494:string)  [unwired: 3 in]
        n294 = Concatenate Strings("abs:" ("string"), w495, w493, w494, w493) -> (w498:string)
        n295 = Enqueue Element(queue=w499, element=w498) -> ()  [unwired: 2 in, 3 out]
      }
      event "ESP_set_t0": Value Change {
        n296 = event-data() -> ()  [unwired: 1 in, 1 out]
        n297 = Current VI's Path() -> (path=w510:path)
        n298 = Strip Path(path=w510) -> (stripped path=w508:path)  [unwired: 1 out]
        n299 = Strip Path(path=w508) -> (stripped path=w507:path)  [unwired: 1 out]
        n300 = local read "ESP_pos"() -> (w509:dbl)
        "ESP_t0" <- w509
        n301 = Number To Fractional String(number=w509) -> (F-format string=w502:string)  [unwired: 3 in]
        n302 = Build Path(base path=w507, name or relative path="t0.txt") -> (appended path=w504:path)
        n303 = Get Date/Time In Seconds() -> (seconds since 1Jan1904=w506:timestamp)
        n304 = Format Date/Time String(time format string (%c)="%Y.%m.%d %H:%M", seconds (now)=w506) -> (date/time string=w503:string)  [unwired: 1 in]
        n305 = Build Array(w503, w502) -> (w501:string[])
        n306 = call-poly <vilib>:"Write Delimited Spreadsheet.vi"("file path (dialog if empty)"=w504, "1D data"=w501, "append to file? (new file:F)"=TRUE ("append to file? (F)")) -> ()  [unwired: 11 in, 2 out]
      }
      event "ESP_opent0file": Value Change {
        n307 = event-data() -> ()  [unwired: 1 in, 6 out]
        n308 = Current VI's Path() -> (path=w514:path)
        n309 = Strip Path(path=w514) -> (stripped path=w513:path)  [unwired: 1 out]
        n310 = Strip Path(path=w513) -> (stripped path=w515:path)  [unwired: 1 out]
        n311 = call <vilib>:"System Exec.vi"("wait until completion? (T)"=FALSE, "working directory"=w515, "command line"="notepad t0.txt") -> ()  [unwired: 5 in, 4 out]
      }
      event "ESP_+", "ESP_-": Value Change {
        n312 = event-data() -> ()  [unwired: 1 in, 6 out]
        n313 = local read "ESP Axis"() -> (w517:i32)
        n314 = Negate(x="ESP_delta") -> (-x=w524:dbl)
        n315 = Select(t="ESP_delta", s="ESP_+", f=w524) -> (s? t:f=w522:dbl)
        n316 = Number To Decimal String(number=w517) -> (decimal integer string=w520:string)  [unwired: 1 in]
        n317 = Number To Fractional String(number=w522) -> (F-format string=w518:string)  [unwired: 3 in]
        n318 = Concatenate Strings("rel:" ("string"), w520, ":" ("string"), w518) -> (w527:string)
        n319 = Enqueue Element(queue=w521, element=w527) -> ()  [unwired: 2 in, 3 out]
      }
      event "ESP_dest": Value Change {
        n320 = event-data() -> ()  [unwired: 1 in, 6 out]
        n321 = local read "ESP_dest"() -> (w531:dbl)
        n322 = local read "ESP_t0"() -> (w530:dbl)
        n323 = call "mm2time.vi"("fs?"=TRUE ("fs[1]/ps[0]"), "Offset (mm)"=w530, "distance (mm)"=w531) -> ("time in fs/ps seconds"=w528:dbl)
        n324 = local write "ESP_dest_t"(w528) -> ()
      }
      event "ESP_dest_t": Value Change {
        n325 = event-data() -> ()  [unwired: 1 in, 1 out]
        n326 = local read "ESP_t0"() -> (w534:dbl)
        n327 = call "time2mm.vi"("fs[1]/ps[0]"=TRUE, "Offset (mm)"=w534, "time"="ESP_dest_t") -> ("position (mm)"=w532:dbl)
        n328 = local write "ESP_dest"(w532) -> ()
      }
      event "load delay table": Value Change {
        n329 = event-data() -> ()  [unwired: 1 in, 6 out]
        n330 = call-poly <vilib>:"Read Delimited Spreadsheet.vi"() -> ("all rows"=w537:string[][], "error out"=w536:errorcluster)  [unwired: 10 in, 4 out]
        n331 = case shown="No Error" w536 {
          tunnel: w537 -> [w538 _]
          frame No Error {
            n332 = local write "waypoints"(w538) -> ()
          }
          frame Error {
          }
        }
      }
      event "mainimg": Cursor Release {
        n333 = event-data() -> ()  [unwired: 1 in, 1 out]
        n334 = Enqueue Element(queue=w540, element="refresh") -> ()  [unwired: 2 in, 3 out]
      }
      event "mirr_init", "mirr_release": Value Change {
        n335 = event-data() -> ()  [unwired: 1 in, 6 out]
        n336 = Flush Queue(queue=w542) -> (queue out=w543:refnum<queue>)  [unwired: 1 in, 2 out]
        n337 = Select(t="init" ("name (unnamed)"), s="mirr_init", f="release" ("name (unnamed)")) -> (s? t:f=w544:string)
        n338 = Enqueue Element(queue=w543, element=w544) -> ()  [unwired: 2 in, 3 out]
      }
      event "mirr_X-", "mirr_X+", "mirr_Y+", "mirr_Y-": Value Change {
        n339 = event-data() -> ()  [unwired: 1 in, 1 out]
        n340 = local read "mirr_X#"() -> (w554:u8)
        n341 = local read "mirr_Y#"() -> (w553:u8)
        n342 = Or(x="mirr_X+", y="mirr_X-") -> (x .or. y?=w555:bool)
        n343 = Or(x="mirr_X-", y="mirr_Y-") -> (x .or. y?=w561:bool)
        n344 = Negate(x="mirr_rel") -> (-x=w560:i32)
        n345 = Select(t=w554, s=w555, f=w553) -> (s? t:f=w552:u8)
        n346 = Select(t=w560, s=w561, f="mirr_rel") -> (s? t:f=w549:i32)
        n347 = Number To Decimal String(number=w552) -> (decimal integer string=w551:string)  [unwired: 1 in]
        n348 = Number To Decimal String(number=w549) -> (decimal integer string=w548:string)  [unwired: 1 in]
        n349 = Concatenate Strings("rel:" ("string"), w551, ":" ("string"), w548) -> (w547:string)
        n350 = Enqueue Element(queue=w563, element=w547) -> ()  [unwired: 2 in, 3 out]
      }
    }
  }
  n351 = while {
    tunnel: w14 -> [w590]
    shift-right: [w584] -> _
    shift-left: _ -> [w583]
    shift-right: [w582] -> _
    shift-left: _ -> [w580]
    shift-right: [w581] -> _
    shift-left: _ -> [w579]
    shift-right: [w576] -> _
    shift-left: 0 -> [w577]
    shift-right: [w575] -> _
    shift-left: _ -> [w574]
    shift-right: [w573] -> _
    shift-left: _ -> [w572]
    tunnel: w23 -> [w571]
    shift-right: [w570] -> _
    shift-left: _ -> [w569]
    shift-right: [w567] -> _
    shift-left: _ -> [w566]
    shift-right: [w565] -> _
    shift-left: _ -> [w564]
    i -> [w568]
    stop <- w578 stop-if-true
    # "cam"
    n352 = Preview Queue Element(queue=w590, timeout in ms (-1)=w577) -> (queue out=w589:refnum<queue>, element=w588:string)  [unwired: 1 in, 2 out]
    n353 = Match Pattern(string=w588, regular expression=":") -> (before substring=w585:string, after substring=w586:string)  [unwired: 1 in, 2 out]
    n354 = case shown="\"idle\", Default" w585 {
      tunnel: w589 -> [w602 w634 w667 w680 _ w768 w798 w863]
      tunnel: w586 -> [_ _ _ _ _ _ _ _]
      tunnel: [w596 w621 w666 w678 w721 w765 w783 w861] -> w584
      tunnel: w583 -> [_ _ w666 w678 w721 w765 w783 w861]
      tunnel: [w601 w635 u64 0 ("Hout") w677 w725 w766 w793 w860] -> w582
      tunnel: [w603 w636 w663 w676 w726 w767 w784 w859] -> w581
      tunnel: w580 -> [_ w638 w665 w677 w728 w770 w795 w860]
      tunnel: w579 -> [_ w637 _ w676 w727 w769 w794 w859]
      tunnel: [_ _ _ TRUE _ _ _ _] -> w578
      tunnel: [_ _ -1 _ _ _ _ -1] -> w576
      tunnel: [w595 w622 _ _ w735 _ _ _] -> w575
      tunnel: w574 -> [w595 w622 _ _ w734 _ _ _]
      tunnel: [w596 w624 w661 w675 w730 w759 w796 w858] -> w573
      tunnel: w572 -> [_ w624 w661 w675 w730 _ w796 w858]
      tunnel: w571 -> [_ _ _ _ _ _ w787 _]
      tunnel: [w593 w619 w660 w673 w688 w756 w790 w857] -> w570
      tunnel: w569 -> [w593 w619 w660 w673 w723 w756 w790 w857]
      tunnel: w568 -> [_ _ _ _ w696 _ _ _]
      tunnel: [w594 w620 w659 w674 w722 w755 w789 w856] -> w567
      tunnel: w566 -> [w594 w620 w659 w674 w695 w755 w789 w856]
      tunnel: [w592 w616 refnum<k21> refnum ("task out") w672 w681 w754 w780 w855] -> w565
      tunnel: w564 -> [_ w616 w658 w672 w681 w754 w781 w855]
      frame "init" {
        w596 = u16[][] []
        n355 = flat-sequence {
          tunnel: [w605] -> w600
          tunnel: [w606] -> w599
          tunnel: [w614] -> w601
          tunnel: [w615] -> w603
          tunnel: w600 -> [w615]
          tunnel: w599 -> [w614]
          frame #0 {
            n356 = local write "cam_con?"(FALSE ("cam_con?")) -> ()
          }
          frame #1 {
            n357 = call "SCInitBoard.vi"("boardnr"="board number") -> ("Hout"=w609:u32, "error out"=w610:errorcluster)  [unwired: 1 in, 1 out]
            n358 = call "SCSetupCamera.vi"("Handle"=w609, "error in (no error)"=w610) -> ("Hout"=w611:u64, "error out"=w612:errorcluster)  [unwired: 1 out]
            n359 = call "SCStopCOC.vi"("error in (no error)"=w612, "Stop mode"=0, "Handle"=w611) -> ("error out"=w605:errorcluster, "Hout"=w606:u64)
          }
          frame #2 {
            n360 = local write "cam_con?"(TRUE ("cam_con?")) -> ()
          }
        }
        n361 = Dequeue Element(queue=w602) -> (queue out=w598:refnum<queue>)  [unwired: 2 in, 3 out]
        n362 = Enqueue Element At Opposite End(queue=w598, element="set") -> ()  [unwired: 2 in, 3 out]
        n363 = call-poly <vilib>:"DAQmx Create Virtual Channel.vi"("lines"=tag "Dev2/port0/line7") -> ("task out"=w592:refnum<k21>)  [unwired: 13 in, 1 out]
      }
      frame "set" {
        n364 = Dequeue Element(queue=w634) -> ()  [unwired: 2 in, 4 out]
        n365 = call "SCStopCOC.vi"("error in (no error)"=w637, "Stop mode"=0, "Handle"=w638) -> ("error out"=w653:errorcluster, "Hout"=w652:u64)
        n366 = Bundle By Name(cluster=cluster{"Delay":dbl, "Exposure ":dbl} {"Delay"=0.0, "Exposure "=0.0} ("Delay and exposure"), "Exposure"="cam_exp") -> (w631:cluster{"Delay":dbl, "Exposure ":dbl})
        n367 = Bundle By Name(cluster=T5 {"Camera type"=0, "Operating mode\nHP & QE / HS & DiCam Pro "=0, "Frame trigger \n(High Performance and QE only)"=0, "Sequence trigger"=0, "Low Light\n(QE only)"=FALSE, "Gain"=FALSE, "Horzontal\nbinning"=0, "Vertical\nbinning "=0, "ROI Left"=1, "ROI Right"=20, "ROI Top"=1, "ROI Bottom"=15} ("Camera controls"), "Operating mode\nHP & QE / HS & DiCam Pro"="Operating mode\nHP & QE / HS & DiCam Pro", "Horzontal\nbinning"="binning", "Vertical\nbinning"="binning", "ROI Left"="ROI Left", "ROI Right"="ROI Right", "ROI Top"="ROI Top", "ROI Bottom"="ROI Bottom", "Gain"="gain", "Frame trigger \n(High Performance and QE only)"="Frame trigger \n(High Performance and QE only)") -> (w648:T5)
        n368 = call "New delay and exposure forma.vi"("Operating mode\nHP & QE / HS & DiCam Pro"="Operating mode\nHP & QE / HS & DiCam Pro", "Delay and exposure"=w631) -> ("Output table"=w649:string)  [unwired: 3 in]
        n369 = call "SCSetCoC.vi"("error in (no error)"=w653, "Delay and exposure table"=w649, "Camera controls"=w648, "Handle"=w652) -> ("error out"=w641:errorcluster, "Hout"=w640:u64)  [unwired: 1 out]
        n370 = call "SCGetImageSize.vi"("Handle"=w640, "error in (no error)"=w641) -> ("Hout"=w639:u64, "error out"=w623:errorcluster, "Horizontal size"=w628:i32, "Vertical size"=w627:i32)  [unwired: 2 out]
        n371 = Greater?(x=w628, y=w627) -> (0:w629:bool)
        n372 = Initialize Array(u16 0 ("dimension size"), w627, w628) -> (w621:u16[][])
        n373 = call "SCRun.vi"("error in (no error)"=w623, "Run mode"=0, "Handle"=w639) -> ("error out"=w636:errorcluster, "Hout"=w635:u64)  [unwired: 1 out]
        n374 = Select(t=w628, s=w629, f=w627) -> (s? t:f=w626:i32)
        n375 = property on="mainimg" class="IntGraph (strict)"("XScale.Maximum"=w626, "YScale.Maximum"=w626) -> ()  [unwired: 2 in, 2 out]
      }
      frame "release" {
        n376 = Dequeue Element(queue=w667) -> (queue out=w654:refnum<queue>)  [unwired: 2 in, 3 out]
        n377 = flat-sequence {
          tunnel: w665 -> [w669]
          tunnel: [w668] -> w662
          tunnel: [w671] -> w663
          tunnel: w662 -> [w671]
          frame #0 {
            n378 = call "SCCloseBoard.vi"("Handle"=w669) -> ("error out"=w668:errorcluster)  [unwired: 1 in, 2 out]
          }
          frame #1 {
            n379 = local write "cam_con?"(FALSE ("cam_con?")) -> ()
          }
        }
        n380 = Enqueue Element(queue=w654, element="suspend") -> ()  [unwired: 2 in, 3 out]
        n381 = call <vilib>:"DAQmx Clear Task.vi"("task in"=w658) -> ()  [unwired: 14 in, 1 out]
      }
      frame "close" {
        n382 = Release Queue(queue=w680) -> ()  [unwired: 2 in, 3 out]
      }
      frame "idle", Default {
        n383 = call "grabimg.vi"("array in"=w721, "error in"=w727, "Hin"=w728) -> ("error out"=w726:errorcluster, "imgdata"=w724:i32[][], "Hout"=w725:u64)  [unwired: 6 in]
        n384 = local read "lower threshold"() -> (w719:i32)
        n385 = case shown="False" "cam_dark?" {
          tunnel: w730 -> [_ w753]
          tunnel: [w750 w752] -> w720
          tunnel: w724 -> [w750 w751]
          frame False {
          }
          frame True {
            n386 = Subtract(x=w751, y=w753) -> (x-y=w752:dbl[][])
          }
        }
        n387 = call "filtr_b.vi"("threshold"=w719, "input array"=w720) -> ("output array"=w711:dbl[][])  [unwired: 9 in]
        n388 = call <vilib>:"High Resolution Relative Seconds.vi"() -> ("relative seconds"=w735:dbl)
        n389 = Subtract(x=w735, y=w734) -> (x-y=w733:dbl)
        n390 = Array Size(array=w711) -> (size(s)=w710:i32[])
        n391 = Reciprocal(x=w733) -> (1/x=→"cam_fps":dbl)
        n392 = Index Array(array=w710) -> (element #1=w705:i32, element #2=w704:i32)  [unwired: 2 in]
        n393 = Subtract(x=w696, y=w695) -> (x-y=w694:i32)
        n394 = Less Or Equal?(x="pics2avg", y=w694) -> (x <= y?=w717:bool)
        n395 = And(x="reset every n pics", y=w717) -> (x .and. y?=w715:bool)
        n396 = Not(x=w715) -> (.not. x?=w714:bool)
        n397 = call-poly <vilib>:"Ramp Pattern.vi"("start"=0.0, "end"=w705, "samples"=w705) -> ("Ramp Pattern"=w700:dbl[])  [unwired: 7 in, 1 out]
        n398 = call-poly <vilib>:"Ramp Pattern.vi"("start"=0.0, "end"=w704, "samples"=w704) -> ("Ramp Pattern"=w701:dbl[])  [unwired: 7 in, 1 out]
        n399 = property on="mainimg" class="IntGraph (strict)"() -> ("CrsrLis"=w693:T4)  [unwired: 2 in, 2 out]
        n400 = And(x="cam_liveavg", y=w714) -> (x .and. y?=w712:bool)
        n401 = case shown="False" w712 {
          tunnel: w711 -> [w740 w746]
          tunnel: [w740 w743] -> w688
          tunnel: w723 -> [_ w748]
          tunnel: w696 -> [w741 _]
          tunnel: [w741 w749] -> w722
          tunnel: w695 -> [_ w749]
          tunnel: w694 -> [_ w742]
          frame False {
          }
          frame True {
            n402 = Multiply(x=w748, y=w742) -> (x*y=w747:dbl[][])
            n403 = Increment(x=w742) -> (x+1=w744:i32)
            n404 = Add(x=w747, y=w746) -> (x+y=w745:dbl[][])
            n405 = Divide(x=w745, y=w744) -> (x/y=w743:dbl[][])
          }
        }
        "mainimg" <- w688
        n406 = Index Array(array=w693) -> (element #1=w691:T6, element #2=w692:T6)  [unwired: 2 in]
        n407 = Unbundle By Name(w691) -> ("Position.X"=w685:dbl, "Position.Y"=w687:dbl)
        n408 = Unbundle By Name(w692) -> ("Position.X"=w689:dbl, "Position.Y"=w690:dbl)
        n409 = Array Max & Min(array=w688) -> (max value=→"max":dbl)  [unwired: 3 out]
        n410 = Subtract(x=w690, y=w687) -> (x-y=w686:dbl)
        n411 = Subtract(x=w689, y=w685) -> (x-y=w684:dbl)
        n412 = Array Subset(array=w688, index (row)=w687, length (row)=w686) -> (w699:dbl[][])  [unwired: 2 in]
        n413 = Array Subset(array=w688, index (col)=w685, length (col)=w684) -> (w697:dbl[][])  [unwired: 2 in]
        n414 = Array Subset(array=w688, index (row)=w687, length (row)=w686, index (col)=w685, length (col)=w684) -> (w683:dbl[][])
        n415 = Transpose 2D Array(2D array=w699) -> (transposed array=w698:dbl[][])
        n416 = Add Array Elements(numeric array=w683) -> (sum=→"sum" →"Waveform Chart":dbl)
        n417 = for {
          tunnel: w697 -> [w737] mode=indexing
          tunnel: [w736] -> w707 mode=indexing
          n418 = Add Array Elements(numeric array=w737) -> (sum=w736:dbl)
        }
        n419 = for {
          tunnel: w698 -> [w739] mode=indexing
          tunnel: [w738] -> w706 mode=indexing
          n420 = Add Array Elements(numeric array=w739) -> (sum=w738:dbl)
        }
        n421 = Bundle("Ramp Pattern"=w701, w706) -> (→"G2 X":cluster{"Ramp Pattern":dbl[], dbl[]})  [unwired: 1 in]
        n422 = Bundle(w707, "Ramp Pattern"=w700) -> (→"G2 Y":cluster{dbl[], "Ramp Pattern":dbl[]})  [unwired: 1 in]
      }
      frame "dark" {
        n423 = Dequeue Element(queue=w768) -> ()  [unwired: 2 in, 4 out]
        n424 = Array Size(array=w765) -> (size(s)=w764:i32[])
        n425 = Index Array(array=w764) -> (element #1=w763:i32, element #2=w762:i32)  [unwired: 2 in]
        n426 = Initialize Array(0.0 ("element"), w763, w762) -> (w760:dbl[][])
        n427 = for {
          N: "dark avg" -> [_]
          tunnel: w770 -> [w778]
          tunnel: w769 -> [w777]
          tunnel: [w776] -> w767
          tunnel: w765 -> [w775]
          tunnel: [w774] -> w766
          shift-right: [w771] -> w758
          shift-left: w760 -> [w772]
          n428 = call "grabimg.vi"("array in"=w775, "error in"=w777, "Hin"=w778) -> ("error out"=w776:errorcluster, "imgdata"=w773:i32[][], "Hout"=w774:u64)  [unwired: 6 in]
          n429 = Add(x=w773, y=w772) -> (x+y=w771:dbl[][])
        }
        n430 = Divide(x=w758, y="dark avg") -> (x/y=w759:dbl[][])
      }
      frame "snap" {
        n431 = Dequeue Element(queue=w798) -> ()  [unwired: 2 in, 4 out]
        n432 = local read "cam_dark?"() -> (w797:bool)
        n433 = local read "cam_avgs"() -> (w792:i32)
        n434 = To Double Precision Float(number=w783) -> (double precision float=w782:dbl[][])
        n435 = Equal To 0?(x="aq.mode") -> (x = 0?=w785:bool)
        n436 = Get Date/Time In Seconds() -> (seconds since 1Jan1904=w788:timestamp)
        n437 = for {
          N: w792 -> [w810]
          shift-right: [w827] -> w793
          shift-left: w795 -> [w829]
          shift-right: [w815] -> w791
          shift-left: w794 -> [w828]
          tunnel: w797 -> [w825]
          tunnel: w796 -> [w824]
          tunnel: w783 -> [w823]
          tunnel: w788 -> [w819]
          tunnel: w785 -> [w803]
          shift-right: [w811] -> w779
          shift-left: w782 -> [w812]
          shift-right: [w801] -> w780
          shift-left: w781 -> [w801]
          i -> [w799]
          stop <- "abort acq." stop-if-true
          n438 = call "grabimg.vi"("array in"=w823, "error in"=w828, "Hin"=w829) -> ("error out"=w815:errorcluster, "imgdata"=w826:i32[][], "Hout"=w827:u64)  [unwired: 6 in]
          n439 = local read "lower threshold"() -> (w806:i32)
          n440 = Increment(x=w799) -> (x+1=w808:i32)
          "acq. imgs" <- w808
          n441 = Get Date/Time In Seconds() -> (seconds since 1Jan1904=w822:timestamp)
          n442 = case shown="True" w825 {
            tunnel: w826 -> [w851 w854]
            tunnel: w824 -> [_ w853]
            tunnel: [w851 w852] -> w805
            frame False {
            }
            frame True {
              n443 = Subtract(x=w854, y=w853) -> (x-y=w852:dbl[][])
            }
          }
          n444 = Divide(x=w808, y=w810) -> (x/y=→"snap_prog":dbl)
          n445 = Subtract(x=w822, y=w819) -> (x-y=w821:dbl)
          n446 = call "filtr_b.vi"("threshold"=w806, "input array"=w805) -> ("output array"=w804:dbl[][])  [unwired: 9 in]
          n447 = Divide(x=w821, y=w799) -> (x/y=w817:dbl)
          n448 = Multiply(x=w817, y=w810) -> (x*y=w820:dbl)
          n449 = Reciprocal(x=w817) -> (1/x=w816:dbl)
          n450 = case shown="True" "count?" {
            tunnel: w804 -> [w842 w844]
            tunnel: "e-size" -> [_ w846]
            tunnel: w806 -> [_ w845]
            tunnel: [w842 w843] -> w802
            frame False {
            }
            frame True {
              n451 = Array Size(array=w844) -> (size(s)=w848:i32[])
              n452 = call "findr.vi"("thresh"=w845, "esize"=w846, "inp array"=w844) -> ("locs"=w847:i32[][])  [unwired: 8 in]
              n453 = Index Array(array=w848) -> (element #1=w850:i32, element #2=w849:i32)  [unwired: 2 in]
              n454 = call "drawe.vi"("Ysize"=w850, "Xsize"=w849, "pos array"=w847) -> ("img out"=w843:i32[][])  [unwired: 8 in]
            }
          }
          n455 = Add(x=w820, y=w819) -> (x+y=→"ETA":timestamp)
          n456 = local write "cam_fps"(w816) -> ()
          n457 = local write "mainimg"(w804) -> ()
          n458 = case shown="True" w803 {
            tunnel: w802 -> [w832 w840]
            tunnel: w812 -> [w834 w839]
            tunnel: [w833 w837] -> w811
            tunnel: [w831 w836] -> w800
            tunnel: w799 -> [w830 w835]
            frame False {
              n459 = Add(x=w832, y=w834) -> (x+y=w833:dbl[][])
              n460 = Increment(x=w830) -> (x+1=w831:i32)
            }
            frame True {
              n461 = Multiply(x=w839, y=w835) -> (x*y=w841:dbl[][])
              n462 = Increment(x=w835) -> (x+1=w836:i32)
              n463 = Add(x=w840, y=w841) -> (x+y=w838:dbl[][])
              n464 = Divide(x=w838, y=w836) -> (x/y=w837:dbl[][])
            }
          }
          "Pics L" <- w800
          n465 = local write "sideimg"(w811) -> ()
        }
        n466 = Enqueue Element(queue=w787, element=w779, error in (no error)=w791) -> (error out=w784:errorcluster)  [unwired: 1 in, 2 out]
      }
      frame "suspend" {
        n467 = Dequeue Element(queue=w863) -> ()  [unwired: 2 in, 4 out]
      }
    }
    "cam_error" <- w581
  }
  n468 = while {
    tunnel: w4 -> [w872]
    shift-right: [w869] -> _
    shift-left: _ -> [w870]
    tunnel: w3 -> [w868]
    shift-right: [w867] -> _
    shift-left: _ -> [w866]
    shift-right: [w864] -> _
    shift-left: _ -> [w865]
    stop <- w871 stop-if-true
    # "mirr"
    n469 = Preview Queue Element(queue=w872, timeout in ms (-1)=w870) -> (queue out=w875:refnum<queue>, element=w876:string)  [unwired: 1 in, 2 out]
    n470 = Match Pattern(string=w876, regular expression=":") -> (before substring=w874:string, after substring=w873:string)  [unwired: 1 in, 2 out]
    n471 = case shown="\"abs\"" w874 {
      tunnel: w875 -> [w911 w921 w936 w940 w943 w948 _]
      tunnel: w873 -> [w905 w922 _ _ _ _ _]
      tunnel: [_ _ _ TRUE _ _ _] -> w871
      tunnel: [_ _ _ _ -1 _ _] -> w869
      tunnel: w868 -> [w878 _ _ _ _ _ _]
      tunnel: [w897 w918 refnum<visa-resource-name> refnum ("VISA resource name out") w938 w942 w947 w953] -> w867
      tunnel: w866 -> [w910 w920 w935 w938 w942 _ w957]
      tunnel: [w882 w917 w934 w937 w941 w946 w952] -> w864
      tunnel: w865 -> [w909 w919 _ w937 w941 _ w956]
      frame "abs" {
        w893 = u8 20 items=["Echo"=55, "Home"=1, "Move Absolute"=20, "Move Relative"=21, "Move at Constant Speed"=22, "Renumber"=2, "Restore Settings"=36, "Stop"=23] ("Command")
        w908 = u8 20 items=["Echo"=55, "Home"=1, "Move Absolute"=20, "Move Relative"=21, "Move at Constant Speed"=22, "Renumber"=2, "Restore Settings"=36, "Stop"=23] ("Command")
        n472 = Dequeue Element(queue=w911) -> ()  [unwired: 2 in, 4 out]
        n473 = Match Pattern(string=w905, regular expression=":") -> (before substring=w895:string, after substring=w881:string)  [unwired: 1 in, 2 out]
        n474 = Equal?(x=w881, y="wait") -> (x = y?=w879:bool)
        n475 = Scan From String(format string="%g_%g", input string=w895) -> (output 1=w890:dbl, output 2=w889:dbl)  [unwired: 4 in, 3 out]
        n476 = local read "mirr_X#"() -> (w892:u8)
        n477 = Bundle("mirr_X#"=w892, "Command"=w908, w890, "Response Count"=1) -> (w904:T7)  [unwired: 1 in]
        n478 = local read "mirr_Y#"() -> (w891:u8)
        n479 = call "Request Command.vi"("error in (no error)"=w909, "Request"=w904, "VISA resource name"=w910) -> ("error out"=w886:errorcluster, "VISA resource name out"=w887:refnum<visa-resource-name>)  [unwired: 5 in, 2 out]
        n480 = Bundle("mirr_Y#"=w891, "Command"=w893, w889, "Response Count"=1) -> (w888:T8)  [unwired: 1 in]
        n481 = call "Request Command.vi"("error in (no error)"=w886, "Request"=w888, "VISA resource name"=w887) -> ("error out"=w884:errorcluster, "VISA resource name out"=w885:refnum<visa-resource-name>)  [unwired: 5 in, 2 out]
        n482 = local read "mirr_X#"() -> (w902:u8)
        n483 = call "zaber_readpos.vi"("error in (no error)"=w884, "axis"=w902, "VISA in"=w885) -> ("error out"=w898:errorcluster, "position"=w903:i32, "VISA out"=w899:refnum<visa-resource-name>)  [unwired: 6 in]
        n484 = local read "mirr_Y#"() -> (w900:u8)
        n485 = local write "mirr_posX"(w903) -> ()
        n486 = call "zaber_readpos.vi"("error in (no error)"=w898, "axis"=w900, "VISA in"=w899) -> ("error out"=w883:errorcluster, "position"=w901:i32, "VISA out"=w897:refnum<visa-resource-name>)  [unwired: 6 in]
        n487 = local write "mirr_posY"(w901) -> ()
        n488 = case shown="True" w879 {
          tunnel: w883 -> [w912 w916]
          tunnel: [w912 w915] -> w882
          tunnel: w878 -> [_ w914]
          frame False {
          }
          frame True {
            n489 = Send Notification(notification=TRUE, notifier=w914, error in (no error)=w916) -> (error out=w915:errorcluster)  [unwired: 1 out]
          }
        }
      }
      frame "rel" {
        w925 = u8 21 items=["Echo"=55, "Home"=1, "Move Absolute"=20, "Move Relative"=21, "Move at Constant Speed"=22, "Renumber"=2, "Restore Settings"=36, "Stop"=23] ("Command")
        n490 = Dequeue Element(queue=w921) -> ()  [unwired: 2 in, 4 out]
        n491 = Match Pattern(string=w922, regular expression=":") -> (before substring=w927:string, after substring=w926:string)  [unwired: 1 in, 2 out]
        n492 = Decimal String To Number(string=w927) -> (number=w929:i32)  [unwired: 2 in, 1 out]
        n493 = Decimal String To Number(string=w926) -> (number=w930:i32)  [unwired: 2 in, 1 out]
        n494 = Bundle(w929, "Command"=w925, w930, "Response Count"=1) -> (w923:T9)  [unwired: 1 in]
        n495 = call "Request Command.vi"("error in (no error)"=w919, "Request"=w923, "VISA resource name"=w920) -> ("error out"=w917:errorcluster, "VISA resource name out"=w918:refnum<visa-resource-name>)  [unwired: 5 in, 2 out]
      }
      frame "release" {
        n496 = Dequeue Element(queue=w936) -> (queue out=w932:refnum<queue>)  [unwired: 2 in, 3 out]
        n497 = Enqueue Element(queue=w932, element="suspend") -> ()  [unwired: 2 in, 3 out]
        n498 = call "Close.vi"("VISA resource name"=w935) -> ("error out"=w934:errorcluster)  [unwired: 9 in, 1 out]
      }
      frame "close" {
        n499 = Release Queue(queue=w940) -> ()  [unwired: 2 in, 3 out]
      }
      frame "suspend" {
        n500 = Dequeue Element(queue=w943) -> ()  [unwired: 2 in, 4 out]
      }
      frame "init" {
        n501 = Dequeue Element(queue=w948) -> ()  [unwired: 2 in, 4 out]
        n502 = call "Initialize.vi"("VISA resource name"="mirr_VISA") -> ("error out"=w946:errorcluster, "VISA resource name out"=w947:refnum<visa-resource-name>)  [unwired: 8 in, 1 out]
      }
      frame "idle", Default {
        n503 = local read "mirr_X#"() -> (w958:u8)
        n504 = call "zaber_readpos.vi"("error in (no error)"=w956, "axis"=w958, "VISA in"=w957) -> ("error out"=w954:errorcluster, "position"=→"mirr_posX":i32, "VISA out"=w955:refnum<visa-resource-name>)  [unwired: 6 in]
        n505 = local read "mirr_Y#"() -> (w951:u8)
        n506 = call "zaber_readpos.vi"("error in (no error)"=w954, "axis"=w951, "VISA in"=w955) -> ("error out"=w952:errorcluster, "position"=→"mirr_posY":i32, "VISA out"=w953:refnum<visa-resource-name>)  [unwired: 6 in]
      }
    }
    "mirr_Error" <- w864
  }
  n507 = while {
    tunnel: w13 -> [w967]
    shift-right: [w965] -> _
    shift-left: _ -> [w963]
    shift-right: [w964] -> _
    shift-left: _ -> [w962]
    shift-right: [w960] -> _
    shift-left: 0 -> [w961]
    tunnel: w3 -> [w959]
    stop <- w966 stop-if-true
    # "ESP"
    n508 = Preview Queue Element(queue=w967, timeout in ms (-1)=w961) -> (queue out=w970:refnum<queue>, element=w971:string)  [unwired: 1 in, 2 out]
    n509 = Match Pattern(string=w971, regular expression=":") -> (before substring=w969:string, after substring=w968:string)  [unwired: 1 in, 2 out]
    n510 = case shown="\"abs\"" w969 {
      tunnel: w970 -> [_ w982 w1000 w1041 w1044 w1051 w1056]
      tunnel: w968 -> [_ w987 w1007 _ _ _ _]
      tunnel: [_ _ _ _ _ TRUE _] -> w966
      tunnel: [w974 w989 w1001 w1039 refnum<visa-resource-name> refnum ("VISA resource name out") w1048 w1055] -> w965
      tunnel: [w973 w990 w999 w1038 w1046 w1049 w1054] -> w964
      tunnel: w963 -> [w978 w992 w1005 w1039 w1047 w1048 _]
      tunnel: w962 -> [w977 w991 w1006 w1038 _ w1049 _]
      tunnel: [_ _ _ -1 _ _ _] -> w960
      tunnel: w959 -> [_ _ w993 _ _ _ _]
      frame "idle", Default {
        n511 = local read "ESP Axis"() -> (w975:i32)
        n512 = local read "ESP_t0"() -> (w981:dbl)
        n513 = call "Read Actual Position.vi"("error in (no error)"=w977, "Axis (1)"=w975, "VISA resource name"=w978) -> ("error out"=w973:errorcluster, "Position (units)"=w976:dbl, "VISA resource name out"=w974:refnum<visa-resource-name>)  [unwired: 2 in]
        "ESP_pos" <- w976
        n514 = call "mm2time.vi"("fs?"=TRUE, "Offset (mm)"=w981, "distance (mm)"=w976) -> ("time in fs/ps seconds"=→"ESP_delay":dbl)
      }
      frame "rel" {
        n515 = Match Pattern(string=w987, regular expression=":") -> (before substring=w986:string, after substring=w985:string)  [unwired: 1 in, 2 out]
        n516 = Dequeue Element(queue=w982) -> ()  [unwired: 2 in, 4 out]
        n517 = Decimal String To Number(string=w986) -> (number=w984:i32)  [unwired: 2 in, 1 out]
        n518 = Fract/Exp String To Number(string=w985) -> (number=w983:dbl)  [unwired: 3 in, 1 out]
        n519 = call "Move Relative.vi"("error in (no error)"=w991, "Position (0 units)"=w983, "Axis (1)"=w984, "VISA resource name"=w992) -> ("error out"=w990:errorcluster, "VISA resource name out"=w989:refnum<visa-resource-name>)  [unwired: 2 in]
      }
      frame "abs" {
        n520 = Dequeue Element(queue=w1000) -> ()  [unwired: 2 in, 4 out]
        n521 = Match Pattern(string=w1007, regular expression=":") -> (before substring=w1008:string, after substring=w997:string)  [unwired: 1 in, 2 out]
        n522 = Match Pattern(string=w997, regular expression=":") -> (before substring=w996:string, after substring=w995:string)  [unwired: 1 in, 2 out]
        n523 = Decimal String To Number(string=w1008) -> (number=w1004:i32)  [unwired: 2 in, 1 out]
        n524 = Fract/Exp String To Number(string=w996) -> (number=w994:dbl)  [unwired: 3 in, 1 out]
        n525 = call "Move Absolute.vi"("error in (no error)"=w1006, "Position (0 units)"=w994, "Axis (1)"=w1004, "VISA resource name"=w1005) -> ("error out"=w1002:errorcluster, "VISA resource name out"=w1003:refnum<visa-resource-name>)  [unwired: 2 in]
        n526 = case shown="\"wait\"" w995 {
          tunnel: w1004 -> [_ w1026]
          tunnel: w1003 -> [w1011 w1028]
          tunnel: w1002 -> [w1010 w1027]
          tunnel: [w1011 w1014] -> w1001
          tunnel: [w1010 w1023] -> w999
          tunnel: w993 -> [_ w1022]
          frame "", Default {
          }
          frame "wait" {
            n527 = while {
              tunnel: w1026 -> [w1037]
              shift-right: [w1034] -> w1025
              shift-left: w1028 -> [w1036]
              shift-right: [w1033] -> w1024
              shift-left: w1027 -> [w1035]
              stop <- w1032 stop-if-true
              n528 = call "Get Axis Motion Status.vi"("error in (no error)"=w1035, "Axis (1)"=w1037, "VISA resource name"=w1036) -> ("error out"=w1033:errorcluster, "Motion Done"=w1032:bool, "VISA resource name out"=w1034:refnum<visa-resource-name>)  [unwired: 2 in]
            }
            n529 = flat-sequence {
              tunnel: w1025 -> [w1031]
              tunnel: w1024 -> [w1030]
              tunnel: [w1031] -> w1017
              tunnel: [w1030] -> w1016
              frame #0 {
                n530 = Wait (ms)(milliseconds to wait=u32 1000) -> ()  [unwired: 1 out]
              }
            }
            n531 = local read "ESP Axis"() -> (w1018:i32)
            n532 = local read "ESP_t0"() -> (w1020:dbl)
            n533 = call "Read Actual Position.vi"("error in (no error)"=w1016, "Axis (1)"=w1018, "VISA resource name"=w1017) -> ("error out"=w1015:errorcluster, "Position (units)"=w1012:dbl, "VISA resource name out"=w1014:refnum<visa-resource-name>)  [unwired: 2 in]
            n534 = call "mm2time.vi"("fs?"=TRUE, "Offset (mm)"=w1020, "distance (mm)"=w1012) -> ("time in fs/ps seconds"=w1013:dbl)
            n535 = local write "ESP_pos"(w1012) -> ()
            n536 = local write "ESP_delay"(w1013) -> ()
            n537 = Send Notification(notification=TRUE, notifier=w1022, error in (no error)=w1015) -> (error out=w1023:errorcluster)  [unwired: 1 out]
          }
        }
      }
      frame "suspend" {
        n538 = Dequeue Element(queue=w1041) -> ()  [unwired: 2 in, 4 out]
      }
      frame "release" {
        n539 = Dequeue Element(queue=w1044) -> (queue out=w1042:refnum<queue>)  [unwired: 2 in, 3 out]
        n540 = call "Close.vi"("VISA resource name"=w1047) -> ("error out"=w1046:errorcluster)  [unwired: 10 in]
        n541 = Enqueue Element(queue=w1042, element="suspend") -> ()  [unwired: 2 in, 3 out]
      }
      frame "close" {
        n542 = Release Queue(queue=w1051) -> ()  [unwired: 2 in, 3 out]
      }
      frame "init" {
        n543 = Dequeue Element(queue=w1056) -> ()  [unwired: 2 in, 4 out]
        n544 = flat-sequence {
          tunnel: [w1059] -> w1053
          tunnel: [w1058] -> w1052
          tunnel: [w1063] -> w1054
          tunnel: [w1064] -> w1055
          tunnel: w1053 -> [w1064]
          tunnel: w1052 -> [w1063]
          frame #0 {
            n545 = local write "ESP_con?"(FALSE ("ESP_con?")) -> ()
          }
          frame #1 {
            n546 = call "Initialize.vi"("VISA resource name"="ESP301 VISA", "Serial Link (RS232)"=enum16{"RS232", "USB"}."USB") -> ("VISA resource name out"=w1059:refnum<visa-resource-name>, "error out"=w1058:errorcluster)  [unwired: 7 in]
          }
          frame #2 {
            n547 = local write "ESP_con?"(TRUE ("ESP_con?")) -> ()
          }
        }
      }
    }
    "error out" <- w964
  }
  n548 = while {
    tunnel: w12 -> [w1073]
    shift-right: [w1071] -> _
    shift-left: _ -> [w1069]
    shift-right: [w1070] -> _
    shift-left: _ -> [w1068]
    shift-right: [w1066] -> _
    shift-left: 0 -> [w1067]
    tunnel: w3 -> [w1065]
    stop <- w1072 stop-if-true
    # "manip"
    n549 = Preview Queue Element(queue=w1073, timeout in ms (-1)=w1067) -> (queue out=w1076:refnum<queue>, element=w1077:string)  [unwired: 1 in, 2 out]
    n550 = Match Pattern(string=w1077, regular expression=":") -> (before substring=w1075:string, after substring=w1074:string)  [unwired: 1 in, 2 out]
    n551 = case shown="\"idle\", Default" w1075 {
      tunnel: w1076 -> [_ w1089 w1116 w1157 w1195 w1201 w1210 w1215]
      tunnel: w1074 -> [_ _ w1103 w1156 _ _ _ _]
      tunnel: [_ _ _ _ _ _ TRUE _] -> w1072
      tunnel: [w1083 w1091 w1095 w1154 w1197 refnum<k5> refnum ("gateway_connection out") w1208 w1214] -> w1071
      tunnel: [w1082 w1090 w1097 w1153 w1196 w1203 w1207 w1213] -> w1070
      tunnel: w1069 -> [w1085 w1093 w1119 w1147 w1197 w1205 w1208 _]
      tunnel: w1068 -> [w1084 w1092 w1118 w1148 w1196 _ w1207 _]
      tunnel: [_ _ _ _ -1 _ _ _] -> w1066
      tunnel: w1065 -> [_ _ w1094 w1150 _ _ _ _]
      frame "idle", Default {
        n552 = call "sp_manip_get_axis_status.vi"("error in"=w1084, "gateway_connection"=w1085) -> ("error out"=w1082:errorcluster, "axis_out"=w1081:T10, "gateway_connection out"=w1083:refnum<k5>)  [unwired: 5 in, 2 out]
        n553 = for {
          tunnel: w1081 -> [w1088] mode=indexing
          tunnel: [w1087] -> w1080 mode=indexing
          tunnel: [w1086] -> w1079 mode=indexing
          n554 = Unbundle By Name(w1088) -> ("Axis_Position"=w1087:dbl, "moving"=w1086:bool)
        }
        "moving?" <- w1079
        n555 = local write "pos"(w1080) -> ()
      }
      frame "stop" {
        n556 = Dequeue Element(queue=w1089) -> ()  [unwired: 2 in, 4 out]
        n557 = call "sp_manip_abort.vi"("error in"=w1092, "gateway_connection"=w1093) -> ("error out"=w1090:errorcluster, "gateway_connection out"=w1091:refnum<k5>)  [unwired: 6 in, 2 out]
      }
      frame "rel" {
        n558 = Dequeue Element(queue=w1116) -> ()  [unwired: 2 in, 4 out]
        n559 = Match Pattern(string=w1103, regular expression=":") -> (before substring=w1102:string, after substring=w1101:string)  [unwired: 1 in, 2 out]
        n560 = Equal?(x=w1101, y="wait") -> (x = y?=w1099:bool)
        n561 = call "sp_manip_get_axis_status.vi"("error in"=w1118, "gateway_connection"=w1119) -> ("error out"=w1121:errorcluster, "axis_out"=w1108:T10, "gateway_connection out"=w1120:refnum<k5>)  [unwired: 5 in, 2 out]
        n562 = Scan From String(format string="%g_%g_%g_%g_%g_%g", input string=w1102) -> (output 1=w1115:dbl, output 2=w1114:dbl, output 3=w1113:dbl, output 4=w1112:dbl, output 5=w1111:dbl, output 6=w1110:dbl)  [unwired: 8 in, 3 out]
        n563 = for {
          tunnel: w1108 -> [w1142] mode=indexing
          tunnel: [w1141] -> w1106 mode=indexing
          tunnel: [w1140] -> w1107 mode=indexing
          n564 = Unbundle By Name(w1142) -> ("Axis_Name"=w1141:string, "Axis_Position"=w1140:dbl)
        }
        n565 = Build Array(w1115, w1114, w1113, w1112, w1111, w1110) -> (w1109:dbl[])
        n566 = Add(x=w1107, y=w1109) -> (x+y=w1105:dbl[])
        n567 = call "sp_manip_start_move.vi"("error in"=w1121, "target positions"=w1105, "axis names"=w1106, "gateway_connection"=w1120) -> ("error out"=w1098:errorcluster, "gateway_connection out"=w1096:refnum<k5>)  [unwired: 4 in, 2 out]
        n568 = case shown="True" w1099 {
          tunnel: w1098 -> [w1122 w1129]
          tunnel: [w1122 w1126] -> w1097
          tunnel: w1096 -> [w1123 w1130]
          tunnel: [w1123 w1128] -> w1095
          tunnel: w1094 -> [_ w1125]
          frame False {
          }
          frame True {
            n569 = while {
              tunnel: w1130 -> [w1134]
              tunnel: w1129 -> [w1133]
              tunnel: [w1132] -> w1128
              tunnel: [w1131] -> w1127
              stop <- w1135 continue-if-true
              n570 = call "sp_manip_get_axis_status.vi"("error in"=w1133, "gateway_connection"=w1134) -> ("error out"=w1131:errorcluster, "axis_out"=w1137:T10, "gateway_connection out"=w1132:refnum<k5>)  [unwired: 5 in, 2 out]
              n571 = for {
                tunnel: w1137 -> [w1139] mode=indexing
                tunnel: [w1138] -> w1136 mode=indexing
                n572 = Unbundle By Name(w1139) -> ("moving"=w1138:bool)
              }
              n573 = Or Array Elements(Boolean array=w1136) -> (logical OR=w1135:bool)
            }
            n574 = Send Notification(notification=TRUE, notifier=w1125, error in (no error)=w1127) -> (error out=w1126:errorcluster)  [unwired: 1 out]
          }
        }
      }
      frame "abs" {
        n575 = Dequeue Element(queue=w1157) -> ()  [unwired: 2 in, 4 out]
        n576 = call "sp_manip_get_axis_status.vi"("error in"=w1148, "gateway_connection"=w1147) -> ("error out"=w1143:errorcluster, "axis_out"=w1146:T10, "gateway_connection out"=w1144:refnum<k5>)  [unwired: 5 in, 2 out]
        n577 = Match Pattern(string=w1156, regular expression=":") -> (before substring=w1160:string, after substring=w1159:string)  [unwired: 1 in, 2 out]
        n578 = Equal?(x=w1159, y="wait") -> (x = y?=w1149:bool)
        n579 = for {
          tunnel: w1146 -> [w1170] mode=indexing
          tunnel: [w1169] -> w1145 mode=indexing
          n580 = Unbundle By Name(w1170) -> ("Axis_Name"=w1169:string)
        }
        n581 = Scan From String(format string="%g_%g_%g_%g_%g_%g", input string=w1160) -> (output 1=w1166:dbl, output 2=w1165:dbl, output 3=w1164:dbl, output 4=w1163:dbl, output 5=w1162:dbl, output 6=w1161:dbl)  [unwired: 8 in, 3 out]
        n582 = Build Array(w1166, w1165, w1164, w1163, w1162, w1161) -> (w1168:dbl[])
        n583 = call "sp_manip_start_move.vi"("error in"=w1143, "target positions"=w1168, "axis names"=w1145, "gateway_connection"=w1144) -> ("error out"=w1152:errorcluster, "gateway_connection out"=w1151:refnum<k5>)  [unwired: 4 in, 2 out]
        n584 = case shown="True" w1149 {
          tunnel: w1152 -> [w1171 w1182]
          tunnel: [w1171 w1181] -> w1153
          tunnel: w1151 -> [w1172 w1183]
          tunnel: [w1172 w1174] -> w1154
          tunnel: w1150 -> [_ w1180]
          frame False {
          }
          frame True {
            n585 = while {
              tunnel: w1183 -> [w1189]
              tunnel: w1182 -> [w1188]
              tunnel: [w1187] -> w1176
              tunnel: [w1186] -> w1175
              stop <- w1190 continue-if-true
              n586 = call "sp_manip_get_axis_status.vi"("error in"=w1188, "gateway_connection"=w1189) -> ("error out"=w1186:errorcluster, "axis_out"=w1192:T10, "gateway_connection out"=w1187:refnum<k5>)  [unwired: 5 in, 2 out]
              n587 = for {
                tunnel: w1192 -> [w1194] mode=indexing
                tunnel: [w1193] -> w1191 mode=indexing
                n588 = Unbundle By Name(w1194) -> ("moving"=w1193:bool)
              }
              n589 = Or Array Elements(Boolean array=w1191) -> (logical OR=w1190:bool)
            }
            n590 = call "sp_manip_get_axis_status.vi"("error in"=w1175, "gateway_connection"=w1176) -> ("error out"=w1173:errorcluster, "axis_out"=w1178:T10, "gateway_connection out"=w1174:refnum<k5>)  [unwired: 5 in, 2 out]
            n591 = for {
              tunnel: w1178 -> [w1185] mode=indexing
              tunnel: [w1184] -> w1177 mode=indexing
              n592 = Unbundle By Name(w1185) -> ("Axis_Position"=w1184:dbl)
            }
            n593 = local write "pos"(w1177) -> ()
            n594 = Send Notification(notification=TRUE, notifier=w1180, error in (no error)=w1173) -> (error out=w1181:errorcluster)  [unwired: 1 out]
          }
        }
      }
      frame "suspend" {
        n595 = Dequeue Element(queue=w1195) -> ()  [unwired: 2 in, 4 out]
      }
      frame "release" {
        n596 = Dequeue Element(queue=w1201) -> (queue out=w1199:refnum<queue>)  [unwired: 2 in, 3 out]
        n597 = call "sp_manip_disconnect.vi"("gateway_connection"=w1205) -> ("error out"=w1204:errorcluster, "gateway_connection_out"=w1206:refnum<k5>)  [unwired: 7 in, 2 out]
        n598 = call "tcp_gateway_close_connection.vi"("error in"=w1204, "server_connection"=w1206) -> ("error out"=w1203:errorcluster)  [unwired: 5 in]
        n599 = Enqueue Element(queue=w1199, element="suspend") -> ()  [unwired: 2 in, 3 out]
      }
      frame "close" {
        n600 = Release Queue(queue=w1210) -> ()  [unwired: 2 in, 3 out]
      }
      frame "init" {
        n601 = Dequeue Element(queue=w1215) -> ()  [unwired: 2 in, 4 out]
        n602 = flat-sequence {
          tunnel: [w1218] -> w1212
          tunnel: [w1217] -> w1211
          tunnel: [w1228] -> w1213
          tunnel: [w1229] -> w1214
          tunnel: w1212 -> [w1229]
          tunnel: w1211 -> [w1228]
          frame #0 {
            n603 = local write "manip_con?"(FALSE ("manip_con?")) -> ()
          }
          frame #1 {
            n604 = call "tcp_gateway_open_connection.vi"() -> ("gateway_connection"=w1221:refnum<k5>, "error out"=w1220:errorcluster)  [unwired: 5 in, 3 out]
            n605 = call "sp_manip_connect.vi"("error in"=w1220, "gateway_connection"=w1221) -> ("error out"=w1217:errorcluster, "axis_out"=w1219:T10, "gateway_connection out"=w1218:refnum<k5>)  [unwired: 5 in, 2 out]
            n606 = for {
              tunnel: w1219 -> [w1226] mode=indexing
              tunnel: [w1225] -> w1222 mode=indexing
              tunnel: [w1224] -> w1223 mode=indexing
              n607 = Unbundle By Name(w1226) -> ("Axis_Name"=w1225:string, "Axis_Position"=w1224:dbl)
            }
            "axis" <- w1222
            "pos" <- w1223
            n608 = local write "dest"(w1223) -> ()
          }
          frame #2 {
            n609 = local write "manip_con?"(TRUE ("manip_con?")) -> ()
          }
        }
      }
    }
    "error out 2" <- w1070
  }
  n610 = while {
    tunnel: w11 -> [w1241]
    shift-right: [w1230] -> _
    shift-left: 0 -> [w1239]
    shift-right: [w1238] -> _
    shift-left: _ -> [w1237]
    shift-right: [w1236] -> _
    shift-left: _ -> [w1235]
    shift-right: [w1234] -> _
    shift-left: u32 0 ("pHandle") -> [w1233]
    tunnel: w9 -> [w1232]
    tunnel: w3 -> [w1231]
    stop <- w1240 stop-if-true
    # "phoib"
    n611 = Preview Queue Element(queue=w1241, timeout in ms (-1)=w1239) -> (queue out=w1244:refnum<queue>, element=w1245:string)  [unwired: 1 in, 2 out]
    n612 = Match Pattern(string=w1245, regular expression=":") -> (before substring=w1243:string, after substring=w1242:string)  [unwired: 1 in, 2 out]
    n613 = case shown="\"idle\", Default" w1243 {
      tunnel: w1244 -> [_ w1298 w1352 w1369 w1387 w1401 w1406 w1411]
      tunnel: w1242 -> [_ _ w1348 _ _ _ _ _]
      tunnel: [_ _ _ _ _ TRUE _ _] -> w1240
      tunnel: [w1255 w1300 w1317 w1372 w1385 w1399 w1405 w1408] -> w1238
      tunnel: w1237 -> [w1266 w1289 w1338 w1374 w1386 w1399 w1405 _]
      tunnel: [w1254 w1299 w1333 w1371 w1384 w1397 w1403 w1407] -> w1236
      tunnel: w1235 -> [w1264 w1288 _ w1373 _ w1397 w1403 _]
      tunnel: [w1252 w1286 w1316 w1370 w1383 w1398 w1404 w1410] -> w1234
      tunnel: w1233 -> [w1252 w1286 w1336 w1370 w1382 w1398 w1404 _]
      tunnel: w1232 -> [w1253 w1279 w1314 _ _ _ _ _]
      tunnel: w1231 -> [_ _ w1332 _ _ _ _ _]
      tunnel: [_ _ _ _ _ _ -1 _] -> w1230
      frame "idle", Default {
        n614 = call "SL2_AD_DLL_Phoibos_GetDeviceState.vi"("dll_path"=w1266, "pHandle_in"=w1252, "dev_type"=DEF_dev_type."devA (analyzer)", "error in"=w1264) -> ("path out"=w1251:path, "state"=→"state":T2, "error out"=w1250:errorcluster)  [unwired: 2 in]
        n615 = for {
          tunnel: w1252 -> [w1273]
          tunnel: w1253 -> [w1271] mode=indexing
          tunnel: [w1270] -> w1263 mode=indexing
          tunnel: [w1269] -> w1255
          shift-right: [w1268] -> w1254
          shift-left: w1250 -> [w1272]
          tunnel: w1251 -> [w1267]
          n616 = call "SL2_AD_DLL_Phoibos_GetVoltage.vi"("error in"=w1272, "voltage_name"=w1271, "pHandle"=w1273, "dll path in"=w1267) -> ("error out"=w1268:errorcluster, "value"=w1270:dbl, "dll path out"=w1269:path)  [unwired: 3 in]
        }
        n617 = Index Array(array=w1263) -> (element #1=→"phoib_I_1":dbl, element #2=→"phoib_I_2":dbl, element #3=→"phoib_I_3":dbl, element #4=→"phoib_I_4":dbl, element #5=→"phoib_I_5":dbl, element #6=→"phoib_I_6":dbl, element #7=→"phoib_I_7":dbl, element #8=→"phoib_I_8":dbl, element #9=→"phoib_I_9":dbl)  [unwired: 9 in]
      }
      frame "set" {
        n618 = Dequeue Element(queue=w1298) -> ()  [unwired: 2 in, 4 out]
        n619 = Multiply(x="ana_voltrange", y=13) -> (x*y=w1295:i32)
        n620 = Add(x="ana_mode", y=w1295) -> (x+y=w1292:i32)
        n621 = Index Array(array=u32[] [251749632, 251749633, 251749634, 251749635, 251749636, 251749637, 251749638, 251749639, 251749640, 251749641, 251749642, 251749643, 251749644, 251749645, 251749646, 251749647, 251749648, 251749649, 251749650, 251749651, 251749652, 251749653, 251749654, 251749655, 251749656, 251749657, 251749658, 251749659, 251749660, 251749661, 251749662, 251749663, 251749664, 251749665, 251749666, 251749667, 251749668, 251749669, 251749670, 251749671, 251749672, 251749673, 251749674, 251749675, 251749676, 251749677, 251749678, 251749679, 251749680, 251749681, 251749682, 251749683, 251749684, 251749685, 251749686, 251749687, 251749688, 251749689, 251749690, 251749691, 251749692, 251749693, 251749694, 251749695, 251749696] ("modeIDs"), index=w1292) -> (element=w1290:u32)
        n622 = Build Array("phoib_I_1s", "phoib_I_2s", "phoib_I_3s", "phoib_I_4s", "phoib_I_5s", "phoib_I_6s", "phoib_I_7s", "phoib_I_8s", "phoib_I_9s") -> (w1278:dbl[])
        n623 = call "SL2_AD_DLL_Phoibos_SetDeviceMode.vi"("pHandle"=w1286, "error in"=w1288, "value"=w1290, "dev_type"=DEF_dev_type."devA (analyzer)", "dll path in"=w1289) -> ("error out"=w1277:errorcluster, "dll path out"=w1287:path)  [unwired: 4 in]
        n624 = for {
          tunnel: w1286 -> [w1306]
          shift-right: [w1313] -> w1300
          shift-left: w1287 -> [w1310]
          tunnel: w1279 -> [w1305] mode=indexing
          tunnel: w1278 -> [w1304] mode=indexing
          shift-right: [w1312] -> w1299
          shift-left: w1277 -> [w1308]
          n625 = call "SL2_AD_DLL_Phoibos_GetVoltageRange.vi"("error in"=w1308, "voltage_name"=w1305, "pHandle"=w1306, "dll path in"=w1310) -> ("error out"=w1307:errorcluster, "min"=w1302:dbl, "max"=w1303:dbl, "dll path out"=w1309:path)  [unwired: 2 in]
          n626 = In Range and Coerce(upper limit=w1303, x=w1304, lower limit=w1302) -> (coerced(x)=w1301:dbl)  [unwired: 1 out]
          n627 = call "SL2_AD_DLL_Phoibos_SetVoltage.vi"("commit"=TRUE, "pHandle"=w1306, "error in"=w1307, "value"=w1301, "voltageName"=w1305, "dll path in"=w1309) -> ("error out"=w1312:errorcluster, "dll path out"=w1313:path)  [unwired: 3 in]
        }
      }
      frame "setsgl" {
        n628 = Dequeue Element(queue=w1352) -> ()  [unwired: 2 in, 4 out]
        n629 = Match Pattern(string=w1348, regular expression=":") -> (before substring=w1341:string, after substring=w1350:string)  [unwired: 1 in, 2 out]
        n630 = Equal?(x=w1350, y="wait") -> ()  [unwired: 1 out]
        n631 = Match Pattern(string=w1341, regular expression=":") -> (before substring=w1315:string, after substring=w1340:string)  [unwired: 1 in, 2 out]
        n632 = Fract/Exp String To Number(string=w1340) -> (number=w1339:dbl)  [unwired: 3 in, 1 out]
        n633 = call "SL2_AD_DLL_Phoibos_GetVoltageRange.vi"("voltage_name"=w1315, "pHandle"=w1336, "dll path in"=w1338) -> ("error out"=w1345:errorcluster, "min"=w1343:dbl, "max"=w1344:dbl, "dll path out"=w1346:path)  [unwired: 3 in]
        n634 = In Range and Coerce(upper limit=w1344, x=w1339, lower limit=w1343) -> (coerced(x)=w1334:dbl)  [unwired: 1 out]
        n635 = call "SL2_AD_DLL_Phoibos_SetVoltage.vi"("commit"=TRUE, "pHandle"=w1336, "error in"=w1345, "value"=w1334, "voltageName"=w1315, "dll path in"=w1346) -> ("error out"=w1335:errorcluster, "dll path out"=w1337:path)  [unwired: 3 in]
        n636 = while {
          tunnel: w1337 -> [w1368]
          tunnel: w1336 -> [w1362]
          tunnel: w1315 -> [w1367]
          tunnel: w1335 -> [w1366]
          tunnel: w1334 -> [w1365]
          tunnel: [w1362] -> w1316
          tunnel: [w1361] -> w1318
          tunnel: [w1360] -> w1320
          stop <- w1363 stop-if-true
          n637 = call "SL2_AD_DLL_Phoibos_GetVoltage.vi"("error in"=w1366, "voltage_name"=w1367, "pHandle"=w1362, "dll path in"=w1368) -> ("error out"=w1360:errorcluster, "value"=w1364:dbl, "dll path out"=w1361:path)  [unwired: 3 in]
          n638 = Equal?(x=w1365, y=w1364) -> (x = y?=w1363:bool)
        }
        n639 = for {
          tunnel: w1316 -> [w1359]
          tunnel: [w1357] -> w1321 mode=indexing
          tunnel: [w1356] -> w1317
          shift-right: [w1355] -> w1319
          shift-left: w1320 -> [w1358]
          tunnel: w1318 -> [w1354]
          tunnel: w1314 -> [w1353] mode=indexing
          n640 = call "SL2_AD_DLL_Phoibos_GetVoltage.vi"("error in"=w1358, "voltage_name"=w1353, "pHandle"=w1359, "dll path in"=w1354) -> ("error out"=w1355:errorcluster, "value"=w1357:dbl, "dll path out"=w1356:path)  [unwired: 3 in]
        }
        n641 = Index Array(array=w1321) -> (element #1=w1322:dbl, element #2=w1323:dbl, element #3=w1324:dbl, element #4=w1325:dbl, element #5=w1326:dbl, element #6=w1330:dbl, element #7=w1327:dbl, element #8=w1328:dbl, element #9=w1329:dbl)  [unwired: 9 in]
        n642 = local write "phoib_I_1"(w1322) -> ()
        n643 = local write "phoib_I_2"(w1323) -> ()
        n644 = local write "phoib_I_3"(w1324) -> ()
        n645 = local write "phoib_I_4"(w1325) -> ()
        n646 = local write "phoib_I_5"(w1326) -> ()
        n647 = local write "phoib_I_6"(w1330) -> ()
        n648 = local write "phoib_I_7"(w1327) -> ()
        n649 = local write "phoib_I_8"(w1328) -> ()
        n650 = local write "phoib_I_9"(w1329) -> ()
        n651 = Send Notification(notification=TRUE, notifier=w1332, error in (no error)=w1319) -> (error out=w1333:errorcluster)  [unwired: 1 out]
      }
      frame "standby" {
        w1375 = T2 0 items=["Off"=-1, "Standby"=0, "On"=1] ("state")
        n652 = Dequeue Element(queue=w1369) -> ()  [unwired: 2 in, 4 out]
        n653 = call "SL2_AD_DLL_Phoibos_SetDeviceState.vi"("pHandle_in"=w1370, "error in"=w1373, "state"=w1375, "dev_type"=DEF_dev_type."devA (analyzer)", "dll_path"=w1374) -> ("error out"=w1371:errorcluster, "path out"=w1372:path)  [unwired: 2 in]
      }
      frame "release" {
        n654 = Dequeue Element(queue=w1387) -> (queue out=w1377:refnum<queue>)  [unwired: 2 in, 3 out]
        n655 = flat-sequence {
          tunnel: w1386 -> [w1388]
          tunnel: w1382 -> [w1389]
          tunnel: [w1392] -> w1381
          tunnel: [w1391] -> w1380
          tunnel: [u32 0] -> w1379
          tunnel: [w1394] -> w1383
          tunnel: [w1395] -> w1384
          tunnel: [w1396] -> w1385
          tunnel: w1381 -> [w1396]
          tunnel: w1380 -> [w1395]
          tunnel: w1379 -> [w1394]
          frame #0 {
            n656 = call "SL2_AD_DLL_Phoibos_Shutdown.vi"("pHandle"=w1389, "dll path in"=w1388) -> ("error out"=w1391:errorcluster, "dll path out"=w1392:path)  [unwired: 4 in]
          }
          frame #1 {
            n657 = local write "phoib_con?"(FALSE ("phoib_con?")) -> ()
          }
        }
        n658 = Enqueue Element(queue=w1377, element="suspend") -> ()  [unwired: 2 in, 3 out]
      }
      frame "close" {
        n659 = Release Queue(queue=w1401) -> ()  [unwired: 2 in, 3 out]
      }
      frame "suspend" {
        n660 = Dequeue Element(queue=w1406) -> ()  [unwired: 2 in, 4 out]
      }
      frame "init" {
        n661 = Dequeue Element(queue=w1411) -> ()  [unwired: 2 in, 4 out]
        n662 = flat-sequence {
          tunnel: [w1418] -> w1409
          tunnel: [w1414] -> w1408
          tunnel: [w1413] -> w1407
          tunnel: [w1426] -> w1410
          tunnel: w1409 -> [w1426]
          frame #0 {
            n663 = local write "phoib_con?"(FALSE ("phoib_con?")) -> ()
          }
          frame #1 {
            w1417 = DEF_dev_type."devA (analyzer)" ("dev_type")
            n664 = call "GetSL2AD_VI_dllPath.vi"() -> ("error"=w1421:errorcluster, "Path"=w1422:path)  [unwired: 9 in, 1 out]
            n665 = call "SL2_AD_DLL_List_Devices.vi"("error in"=w1421, "dev_type"=w1417, "dll path in"=w1422) -> ("error out"=w1415:errorcluster, "devices"=w1424:string[], "dll path out"=w1416:path)  [unwired: 2 in]
            n666 = Index Array(array=w1424) -> (element=w1423:string)  [unwired: 1 in]
            n667 = call "SL2_AD_DLL_Phoibos_Initialize.vi"("error in"=w1415, "analyzerId"=w1423, "dll_path"=w1416) -> ("error out"=w1419:errorcluster, "pHandle"=w1418:u32, "path out"=w1420:path)  [unwired: 2 in]
            n668 = call "SL2_AD_DLL_Phoibos_ListDeviceModes.vi"("dll path in"=w1420, "dev_type"=w1417, "pHandle"=w1418, "error in"=w1419) -> ("dll path out"=w1414:path, "error out"=w1413:errorcluster)  [unwired: 1 in, 2 out]
          }
          frame #2 {
            n669 = local write "phoib_con?"(TRUE ("phoib_con?")) -> ()
          }
        }
      }
    }
    "phoib_error" <- w1236
  }
